vi "FeedbackDecode_PickROI_Adv.vi"(3 "RespStrRef":refnum<vi>) -> ()   [LabVIEW 2020]
uses:
  <vilib>/Utility/miscctls.llb/LVPoint32TypeDef.ctl
  FeedbackDecode_Globals.vi
  <vilib>/imath/engines/lvmath2/RunTimeEngine/IndexRead/NIMS M($,S).vi
  <instcachedir>/0/NIMS M($,S)_3E5749BBB62E49528D4765A77F1F6D98.lvgen/NIMS M($,S)_3E5749BBB62E49528D4765A77F1F6D98_000.vi
  <vilib>/imath/engines/lvmath2/RunTimeEngine/IndexRead/NIMS V(S).vi
  <instcachedir>/0/NIMS V(S)_0488751826AF41519A22953C041130DC.lvgen/NIMS V(S)_0488751826AF41519A22953C041130DC_000.vi
  <vilib>/imath/engines/lvmath2/RunTimeEngine/BuiltInFunctions/abs/NIMS_abs(signed).vi
  <instcachedir>/0/NIMS_abs(signed)_C4FCB8E6058B49B797C7C8D53CA5F6EC.lvgen/NIMS_abs(signed)_C4FCB8E6058B49B797C7C8D53CA5F6EC_001.vi
  <vilib>/imath/engines/lvmath2/RunTimeEngine/IndexReplace/NIMS M($,S)=V.vi
  <instcachedir>/0/NIMS M($,S)=V_85A28EB895514E96A13A10261726EE3A.lvgen/NIMS M($,S)=V_85A28EB895514E96A13A10261726EE3A_001.vi
  <vilib>/imath/engines/lvmath2/RunTimeEngine/ErrorHandling/NIMS_Create Error From Enums.vi
  <vilib>/imath/engines/lvmath2/RunTimeEngine/BuiltInFunctions/sum/NIMS_sum(GM,Sca).vi
  <instcachedir>/0/NIMS_sum(GM,Sca)_BFF867FCA20B40888962313BF0DBA2C0.lvgen/NIMS_sum(GM,Sca)_BFF867FCA20B40888962313BF0DBA2C0_001.vi
  <vilib>/imath/engines/lvmath2/RunTimeEngine/BuiltInFunctions/min/1 input/NIMS_min(RV).vi
  <instcachedir>/0/NIMS_min(RV)_EE2DD3E2888846108C5160A664B67832.lvgen/NIMS_min(RV)_EE2DD3E2888846108C5160A664B67832_000.vi
  <vilib>/imath/engines/lvmath2/RunTimeEngine/NodeEndStatement/NIMS_NodeEndStatement_Output.vi
  <instcachedir>/0/NIMS_NodeEndStatement_Output_53EC0D466D134D7ABD903AC30B43404B.lvgen/NIMS_NodeEndStatement_Output_53EC0D466D134D7ABD903AC30B43404B_010.vi
  <vilib>/imath/engines/lvmath2/RunTimeEngine/ErrorHandling/NIMS_Finalize Error.vi
panel:
  out "RegionStr":string
  out "SensorStr":string
  out "Description_array":string[](array[string])
  out "CursClck":dbl[](array[numeric])
  in  "Advance":bool
  out "StepAdvnc":dbl
  out "Perception_array":string[](array[string])
  out "Sensor_array":string[][](array[string])
  out "Region_array":string[][](array[string])
  out "Y_array":dbl[][](array[numeric])
  out "X_array":dbl[][](array[numeric])
  out "Sensor":string[](array[string])
  out "Region":string[](array[string])
  out "Xcoord":dbl[](array[numeric])
  out "Ycoord":dbl[](array[numeric])
  out "Palette":u32[](array[colorbox])=[16711680, 15697664, 16772882, 8584960, 61382, 14847, 11534591]
  out "CrcColor":u32=16711680
  out "PPath2":path=path "C:/Users/Administrator/Code/Tasks/FeedbackDecode/resources/RightHand_region_colored.jpg"
  in  "DscrptnBtns":T1
  in  "ClearRsp":bool
  in  "PerceptBtns":T2
  out "PickROIStr":string
  in  "Array 4":string[][](array[string])
  out "RegionStr":string[][](array[string])=[["G1", "1", "231", "255", "231", "T1", "", ""], ["G2", "2", "201", "254", "200", "T2", "", ""], ["G3", "3", "211", "235", "211", "T3", "", ""], ["G4", "4", "188", "236", "188", "T4", "", ""], ["G5", "5", "141", "235", "141", "T5", "", ""], ["G6", "6", "164", "235", "165", "T6", "", ""], ["G7", "7", "117", "234", "117", "P1", "", ""], ["G8", "8", "70", "235", "70", "P6", "", ""], ["G9", "9", "94", "235", "94", "P9", "", ""], ["G10", "10", "46", "235", "47", "P7", "", ""], ["G11", "11", "3", "235", "3", "P8", "", ""], ["G12", "12", "23", "236", "24", "P10", "", ""], ["R1", "13", "248", "200", "200", "I1", "", ""], ["R2", "14", "248", "180", "181", "I2", "", ""], ["R3", "15", "248", "150", "151", "I3", "", ""], ["R4", "16", "248", "120", "121", "I4", "", ""], ["R5", "17", "248", "100", "100", "I5", "", ""], ["R6", "18", "248", "80", "80", "I6", "", ""], ["R7", "19", "248", "60", "61", "I7", "", ""], ["R8", "20", "248", "30", "29", "I8", "", ""], ["R9", "21", "247", "2", "2", "P2", "", ""], ["O1", "22", "243", "210", "195", "M1", "", ""], ["O2", "23", "244", "194", "171", "M2", "", ""], ["O3", "24", "243", "178", "145", "M3", "", ""], ["O4", "25", "244", "162", "122", "M4", "", ""], ["O5", "26", "243", "145", "98", "M5", "", ""], ["O6", "27", "244", "129", "74", "M6", "", ""], ["O7", "28", "243", "113", "48", "M7", "", ""], ["O8", "29", "243", "97", "24", "M8", "", ""], ["O9", "30", "243", "80", "0", "P3", "", ""], ["Y1", "31", "232", "225", "209", "R1", "", ""], ["Y2", "32", "232", "218", "187", "R2", "", ""], ["Y3", "33", "232", "210", "163", "R3", "", ""], ["Y4", "34", "230", "205", "138", "R4", "", ""], ["Y5", "35", "233", "196", "116", "R5", "", ""], ["Y6", "36", "232", "187", "93", "R6", "", ""], ["Y7", "37", "233", "181", "71", "R7", "", ""], ["Y8", "38", "232", "173", "47", "R8", "", ""], ["Y9", "39", "232", "159", "0", "P4", "", ""], ["YG1", "40", "213", "232", "186", "L1", "", ""], ["YG2", "41", "202", "232", "162", "L2", "", ""], ["YG3", "42", "193", "232", "139", "L3", "", ""], ["YG4", "43", "182", "232", "117", "L4", "", ""], ["YG5", "44", "171", "232", "93", "L5", "", ""], ["YG6", "45", "161", "231", "70", "L6", "", ""], ["YG7", "46", "152", "232", "47", "L7", "", ""], ["YG8", "47", "142", "232", "23", "L8", "", ""], ["YG9", "48", "130", "234", "0", "P5", "", ""], ["P1", "49", "250", "227", "253", "DT1", "", ""], ["P2", "50", "245", "203", "253", "DT2", "", ""], ["P3", "51", "241", "177", "253", "DT3", "", ""], ["P4", "52", "238", "152", "253", "DT4", "", ""], ["P5", "53", "235", "126", "253", "DT5", "", ""], ["P6", "54", "230", "101", "253", "DT6", "", ""], ["P7", "55", "227", "76", "253", "D1", "", ""], ["P8", "56", "223", "50", "253", "D6", "", ""], ["P9", "57", "220", "25", "253", "D9", "", ""], ["P10", "58", "215", "0", "254", "D7", "", ""], ["P11", "59", "167", "0", "254", "D8", "", ""], ["P12", "60", "188", "52", "255", "D10", "", ""], ["BG1", "61", "204", "240", "234", "DI1", "", ""], ["BG2", "62", "168", "240", "226", "DI2", "", ""], ["BG3", "63", "144", "240", "221", "DI3", "", ""], ["BG4", "64", "120", "240", "216", "DI4", "", ""], ["BG5", "65", "96", "240", "211", "DI5", "", ""], ["BG6", "66", "72", "240", "206", "DI6", "", ""], ["BG7", "67", "48", "240", "202", "DI7", "", ""], ["BG8", "68", "24", "240", "197", "DI8", "", ""], ["BG9", "69", "0", "240", "192", "D2", "", ""], ["LB1", "70", "186", "229", "232", "DM1", "", ""], ["LB2", "71", "163", "228", "232", "DM2", "", ""], ["LB3", "72", "139", "226", "232", "DM3", "", ""], ["LB4", "73", "116", "225", "232", "DM4", "", ""], ["LB5", "74", "93", "223", "232", "DM5", "", ""], ["LB6", "75", "70", "222", "232", "DM6", "", ""], ["LB7", "76", "46", "220", "232", "DM7", "", ""], ["LB8", "77", "23", "218", "232", "DM8", "", ""], ["LB9", "78", "0", "217", "232", "D3", "", ""], ["B1", "79", "204", "224", "255", "DR1", "", ""], ["B2", "80", "179", "208", "255", "DR2", "", ""], ["B3", "81", "153", "192", "255", "DR3", "", ""], ["B4", "82", "127", "177", "255", "DR4", "", ""], ["B5", "83", "103", "161", "255", "DR5", "", ""], ["B6", "84", "76", "145", "255", "DR6", "", ""], ["B7", "85", "52", "129", "255", "DR7", "", ""], ["B8", "86", "25", "113", "255", "DR8", "", ""], ["B9", "87", "0", "96", "255", "D4", "", ""], ["BP1", "88", "230", "230", "255", "DL1", "", ""], ["BP2", "89", "180", "179", "255", "DL2", "", ""], ["BP3", "90", "155", "153", "255", "DL3", "", ""], ["BP4", "91", "130", "127", "255", "DL4", "", ""], ["BP5", "92", "105", "103", "255", "DL5", "", ""], ["BP6", "93", "79", "76", "255", "DL6", "", ""], ["BP7", "94", "54", "52", "255", "DL7", "", ""], ["BP8", "95", "29", "25", "255", "DL8", "", ""], ["BP9", "96", "6", "0", "255", "D5", "", ""]]
  in  "Array 3":dbl[][](array[numeric])
  out "RGB 2":dbl[](array[numeric])=[92.0, 223.0, 233.0]
  out "RGBtbl 2":dbl[][](array[numeric])=[[231.0, 255.0, 231.0], [201.0, 254.0, 200.0], [211.0, 235.0, 211.0], [188.0, 236.0, 188.0], [141.0, 235.0, 141.0], [164.0, 235.0, 165.0], [117.0, 234.0, 117.0], [70.0, 235.0, 70.0], [94.0, 235.0, 94.0], [46.0, 235.0, 47.0], [3.0, 235.0, 3.0], [23.0, 236.0, 24.0], [248.0, 200.0, 200.0], [248.0, 180.0, 181.0], [248.0, 150.0, 151.0], [248.0, 120.0, 121.0], [248.0, 100.0, 100.0], [248.0, 80.0, 80.0], [248.0, 60.0, 61.0], [248.0, 30.0, 29.0], [247.0, 2.0, 2.0], [243.0, 210.0, 195.0], [244.0, 194.0, 171.0], [243.0, 178.0, 145.0], [244.0, 162.0, 122.0], [243.0, 145.0, 98.0], [244.0, 129.0, 74.0], [243.0, 113.0, 48.0], [243.0, 97.0, 24.0], [243.0, 80.0, 0.0], [232.0, 225.0, 209.0], [232.0, 218.0, 187.0], [232.0, 210.0, 163.0], [230.0, 205.0, 138.0], [233.0, 196.0, 116.0], [232.0, 187.0, 93.0], [233.0, 181.0, 71.0], [232.0, 173.0, 47.0], [232.0, 159.0, 0.0], [213.0, 232.0, 186.0], [202.0, 232.0, 162.0], [193.0, 232.0, 139.0], [182.0, 232.0, 117.0], [171.0, 232.0, 93.0], [161.0, 231.0, 70.0], [152.0, 232.0, 47.0], [142.0, 232.0, 23.0], [130.0, 234.0, 0.0], [250.0, 227.0, 253.0], [245.0, 203.0, 253.0], [241.0, 177.0, 253.0], [238.0, 152.0, 253.0], [235.0, 126.0, 253.0], [230.0, 101.0, 253.0], [227.0, 76.0, 253.0], [223.0, 50.0, 253.0], [220.0, 25.0, 253.0], [215.0, 0.0, 254.0], [167.0, 0.0, 254.0], [188.0, 52.0, 255.0], [204.0, 240.0, 234.0], [168.0, 240.0, 226.0], [144.0, 240.0, 221.0], [120.0, 240.0, 216.0], [96.0, 240.0, 211.0], [72.0, 240.0, 206.0], [48.0, 240.0, 202.0], [24.0, 240.0, 197.0], [0.0, 240.0, 192.0], [186.0, 229.0, 232.0], [163.0, 228.0, 232.0], [139.0, 226.0, 232.0], [116.0, 225.0, 232.0], [93.0, 223.0, 232.0], [70.0, 222.0, 232.0], [46.0, 220.0, 232.0], [23.0, 218.0, 232.0], [0.0, 217.0, 232.0], [204.0, 224.0, 255.0], [179.0, 208.0, 255.0], [153.0, 192.0, 255.0], [127.0, 177.0, 255.0], [103.0, 161.0, 255.0], [76.0, 145.0, 255.0], [52.0, 129.0, 255.0], [25.0, 113.0, 255.0], [0.0, 96.0, 255.0], [230.0, 230.0, 255.0], [180.0, 179.0, 255.0], [155.0, 153.0, 255.0], [130.0, 127.0, 255.0], [105.0, 103.0, 255.0], [79.0, 76.0, 255.0], [54.0, 52.0, 255.0], [29.0, 25.0, 255.0], [6.0, 0.0, 255.0]]
  out "Resample 2":bool=TRUE
  out "Count 2":i32
  out "ErMsg 2":bool
  out "2D Picture 2":picture
  out "Coords":T3={"Horizontal"=176, "Vertical"=80}
  out "Output Color":u32(colorbox)=6086633
  in  "Abort":bool
  out "Click":bool
  out "RGBtbl":dbl[][](array[numeric])=[[236.0, 28.0, 36.0], [216.0, 207.0, 255.0], [249.0, 136.0, 49.0], [165.0, 255.0, 153.0], [249.0, 189.0, 49.0], [236.0, 236.0, 28.0], [52.0, 28.0, 236.0], [170.0, 28.0, 236.0], [236.0, 28.0, 174.0], [255.0, 170.0, 230.0], [140.0, 255.0, 251.0], [27.0, 234.0, 189.0], [25.0, 178.0, 89.0]]
  in  "Array 2":dbl[][](array[numeric])
  out "SensStr":string[][](array[string])=[["Red", "1", "236", "28", "36", "thumb_distal"], ["Lavender", "2", "216", "207", "255", "thumb_distal"], ["Orange", "3", "249", "136", "49", "palm_back"], ["LGreen", "4", "165", "255", "153", "palm_side"], ["Gold", "5", "249", "189", "49", "palm_thumb"], ["Yellow", "6", "236", "236", "28", "palm_pinky"], ["Blue", "7", "52", "28", "236", "pinky_distal"], ["Purple", "8", "170", "28", "236", "ring_distal"], ["Magenta", "9", "236", "28", "174", "middle_distal"], ["Pink", "10", "255", "170", "230", "index_distal"], ["LBlue", "11", "140", "255", "251", "index_medial"], ["BGreen", "12", "27", "234", "189", "thumb_distal"], ["Green", "13", "25", "178", "89", "thumb_medial"]]
  in  "Array":string[][](array[string])
  out "ErMsg":bool
  out "Count":i32=5
  out "Resample":bool
  out "RGB":dbl[](array[numeric])=[255.0, 255.0, 255.0]
  out "2D Picture":picture
  in  "Submit":bool
  # "1. Click on the region(s) where the sensation occurs :"
  # "2. Describe the sensation (choose one):"
  # "3. Choose between each pair:"
  # "4. Describe another \nsensation (optional):"
  # "5. Submit response:"
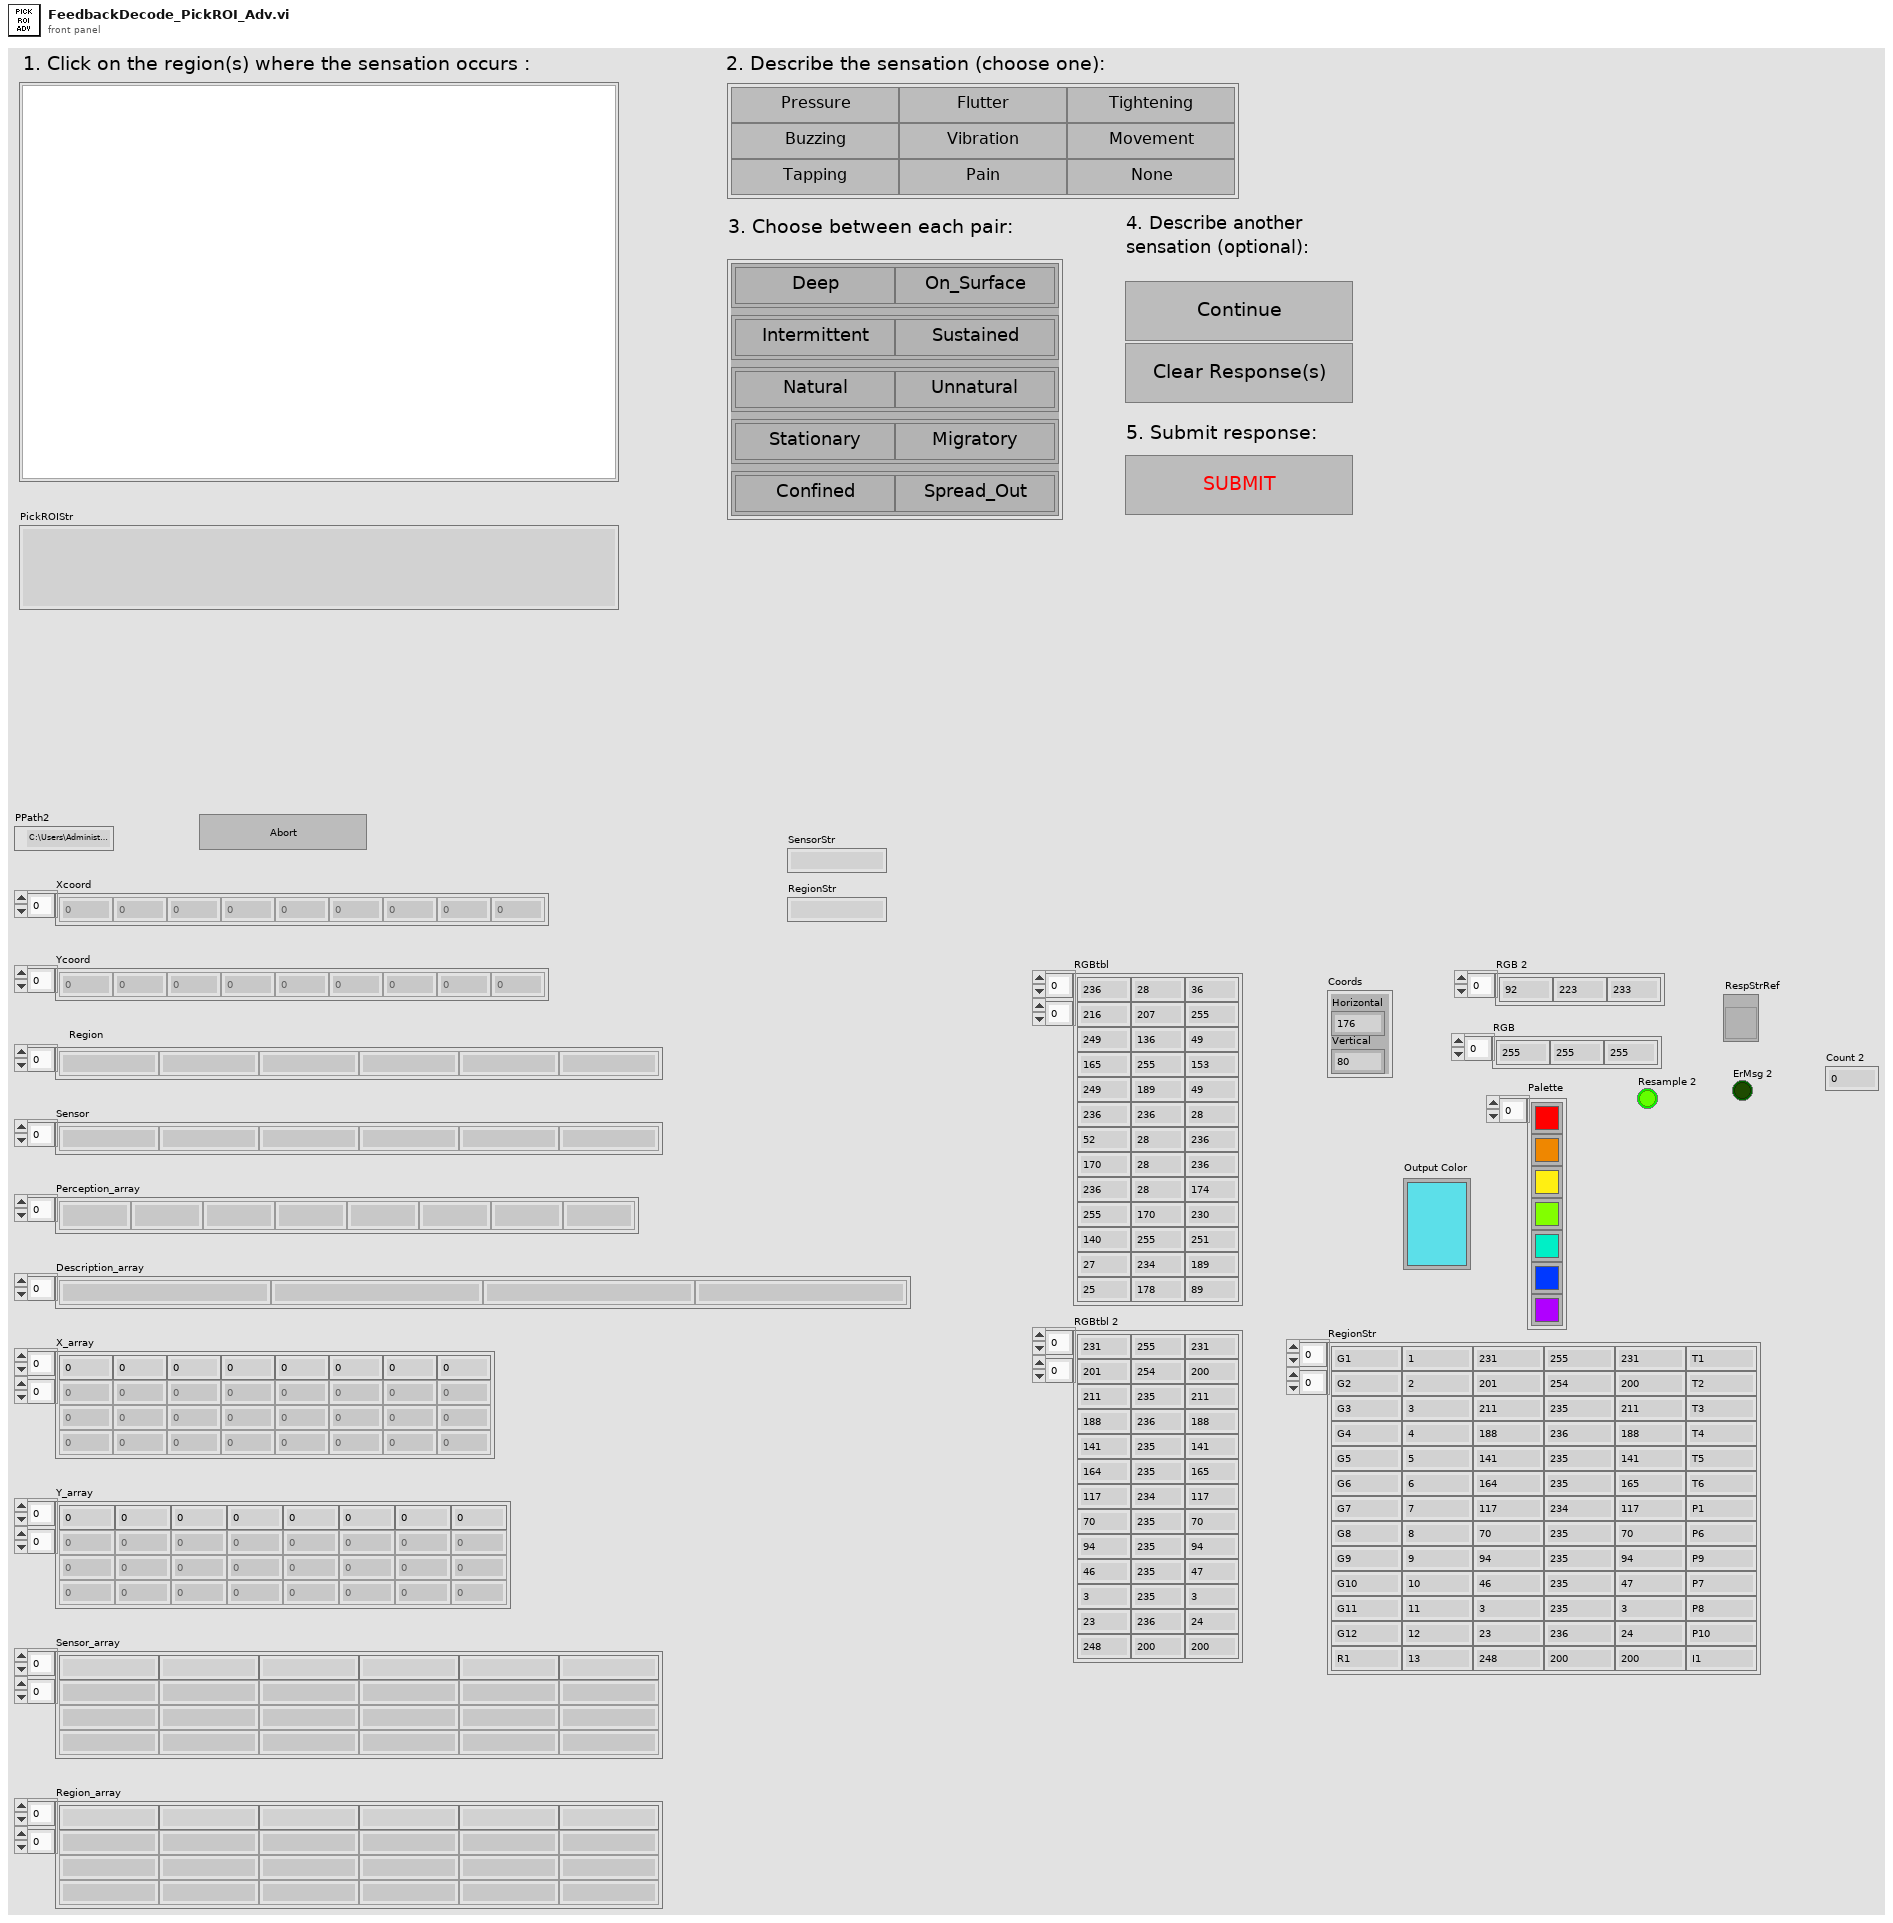
[diagram p1: front panel]
types:
  T1 = cluster{"2afc 3":cluster{"Stationary":bool, "Migratory":bool}, "2afc 2":cluster{"Natural":bool, "Unnatural":bool}, "2afc 4":cluster{"Confined":bool, "Spread":bool}, "2afc 1":cluster{"Intermittent":bool, "Sustained":bool}, "2afc 0":cluster{"Deep":bool, "Surface":bool}}
  T2 = cluster{"Buzzing":bool, "Pressure":bool, "Tapping":bool, "None":bool, "Flutter":bool, "Vibration":bool, "Pain":bool, "Tightening":bool, "Movement":bool}
  T3 = typedef "LVPoint32TypeDef.ctl" = cluster{"Horizontal":i32, "Vertical":i32}
  T4 = cluster{"Motion":bool, "Pressure":bool, "Tapping":bool, "None":bool, "Flutter":bool, "Vibration":bool, "Pain":bool, "Tightening":bool, "Movement":bool}
  T5 = typedef "imagedata.ctl" = cluster{"image type":i32, "image depth":i32, "image":u8[], "mask":u8[], "colors":u32[], "Rectangle":cluster{"left":i16, "top":i16, "right":i16, "bottom":i16}}
  T6 = typedef "LVPositionTypeDef.ctl" = cluster{"Left":i32, "Top":i32}
  T7 = enum32{"Invalid", "Standard", "Closed", "Hidden", "Minimized", "Maximized"}
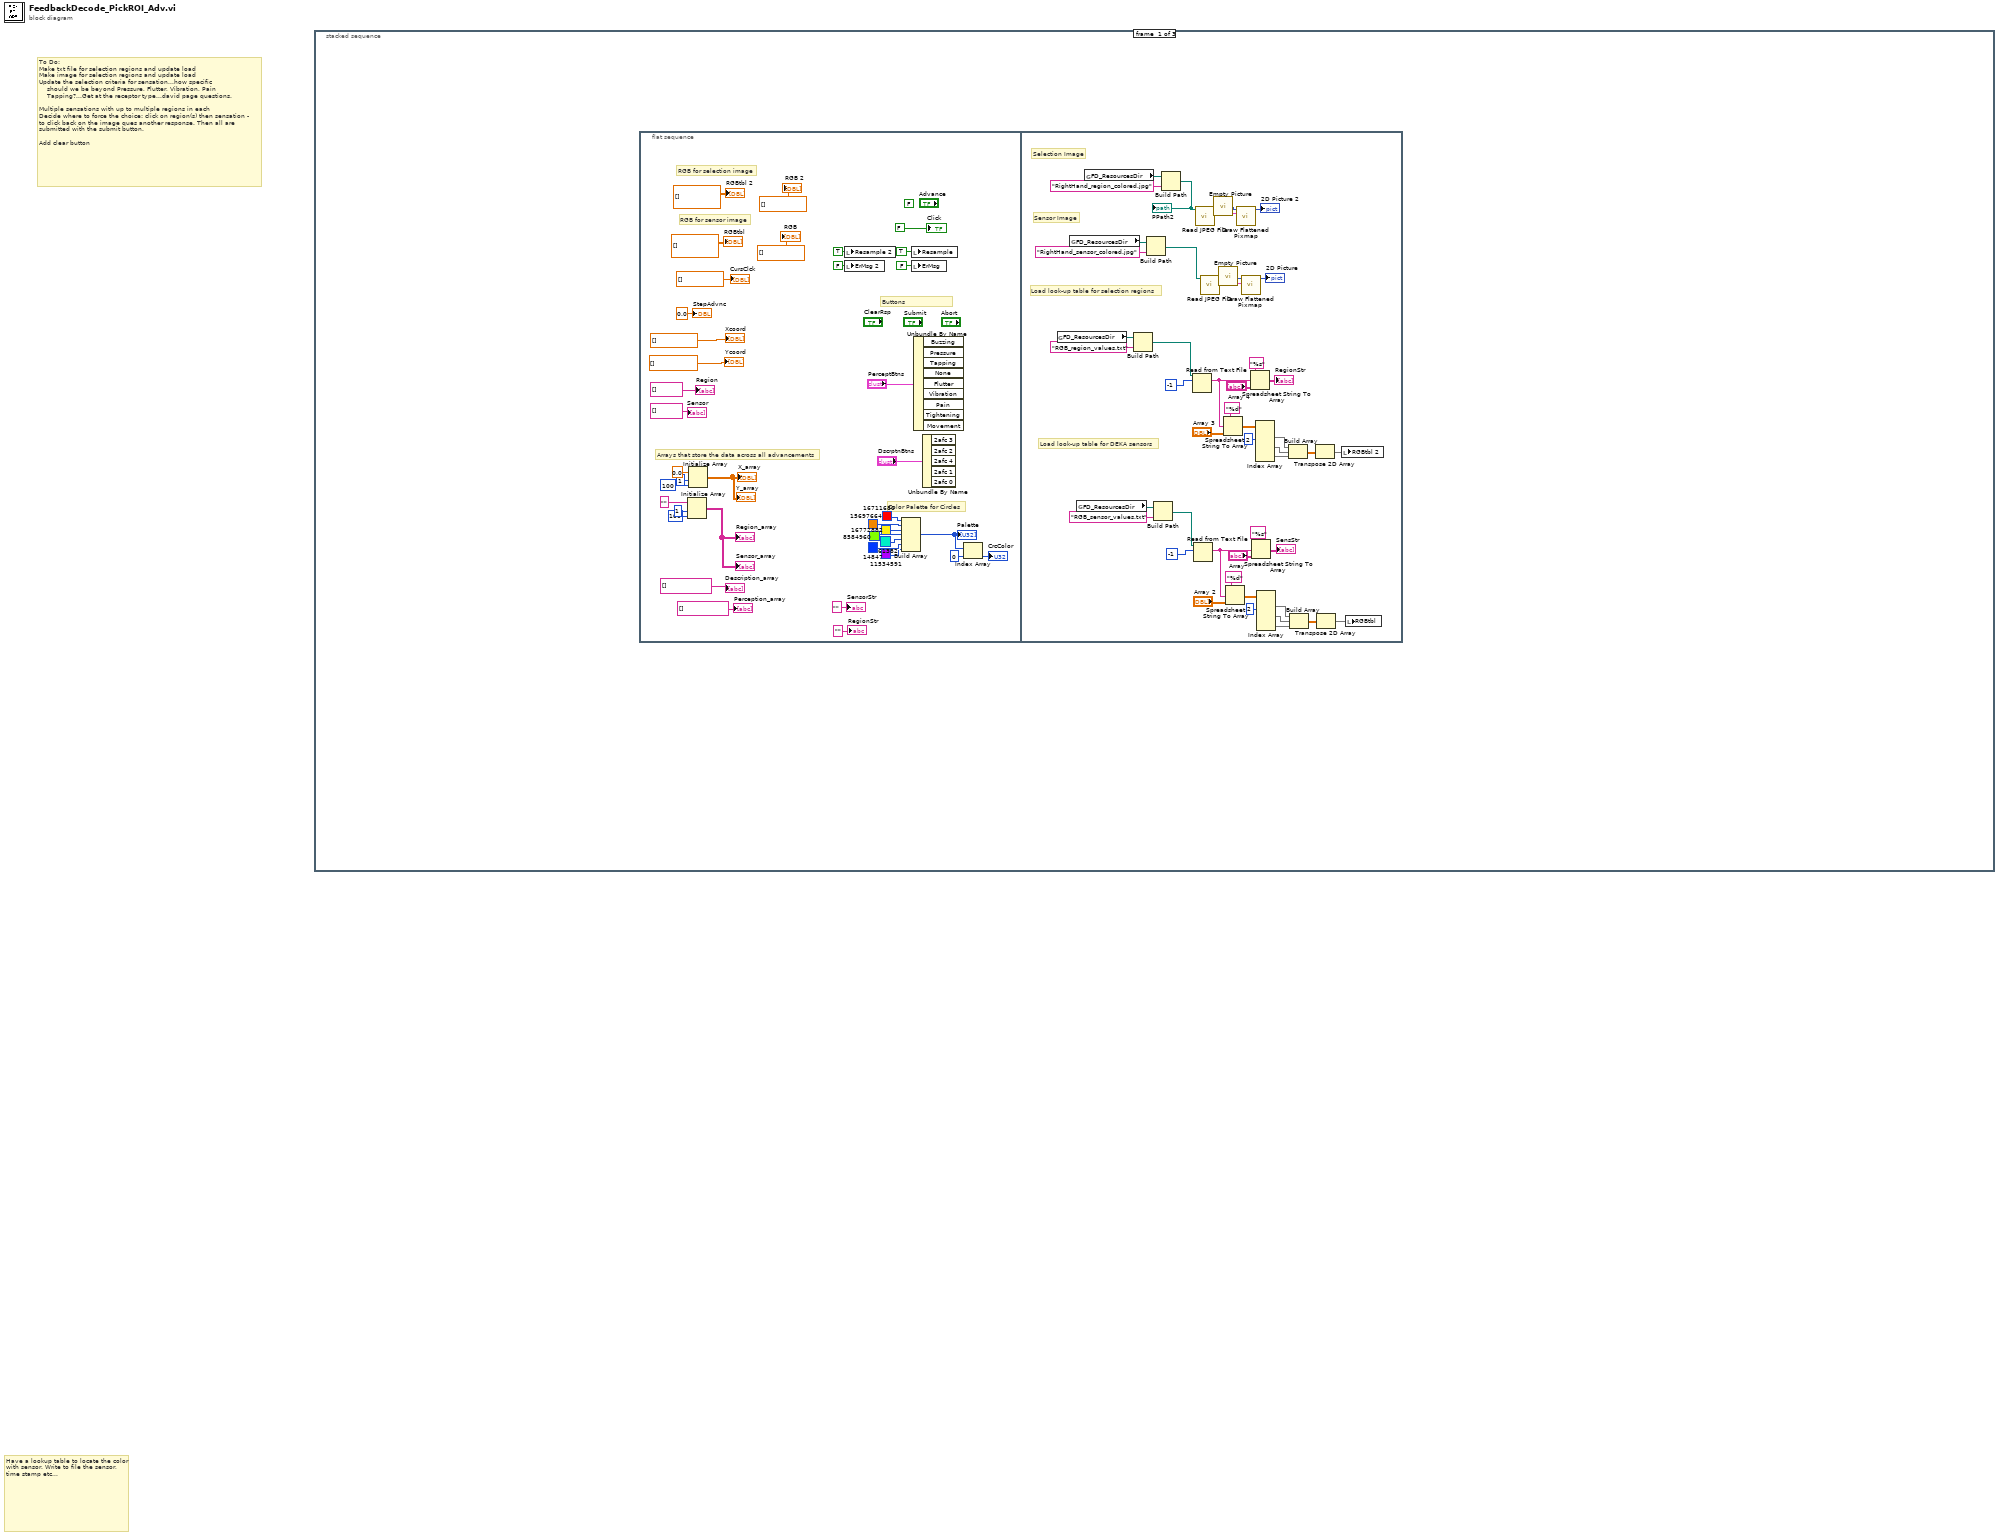
[diagram p0: block diagram]
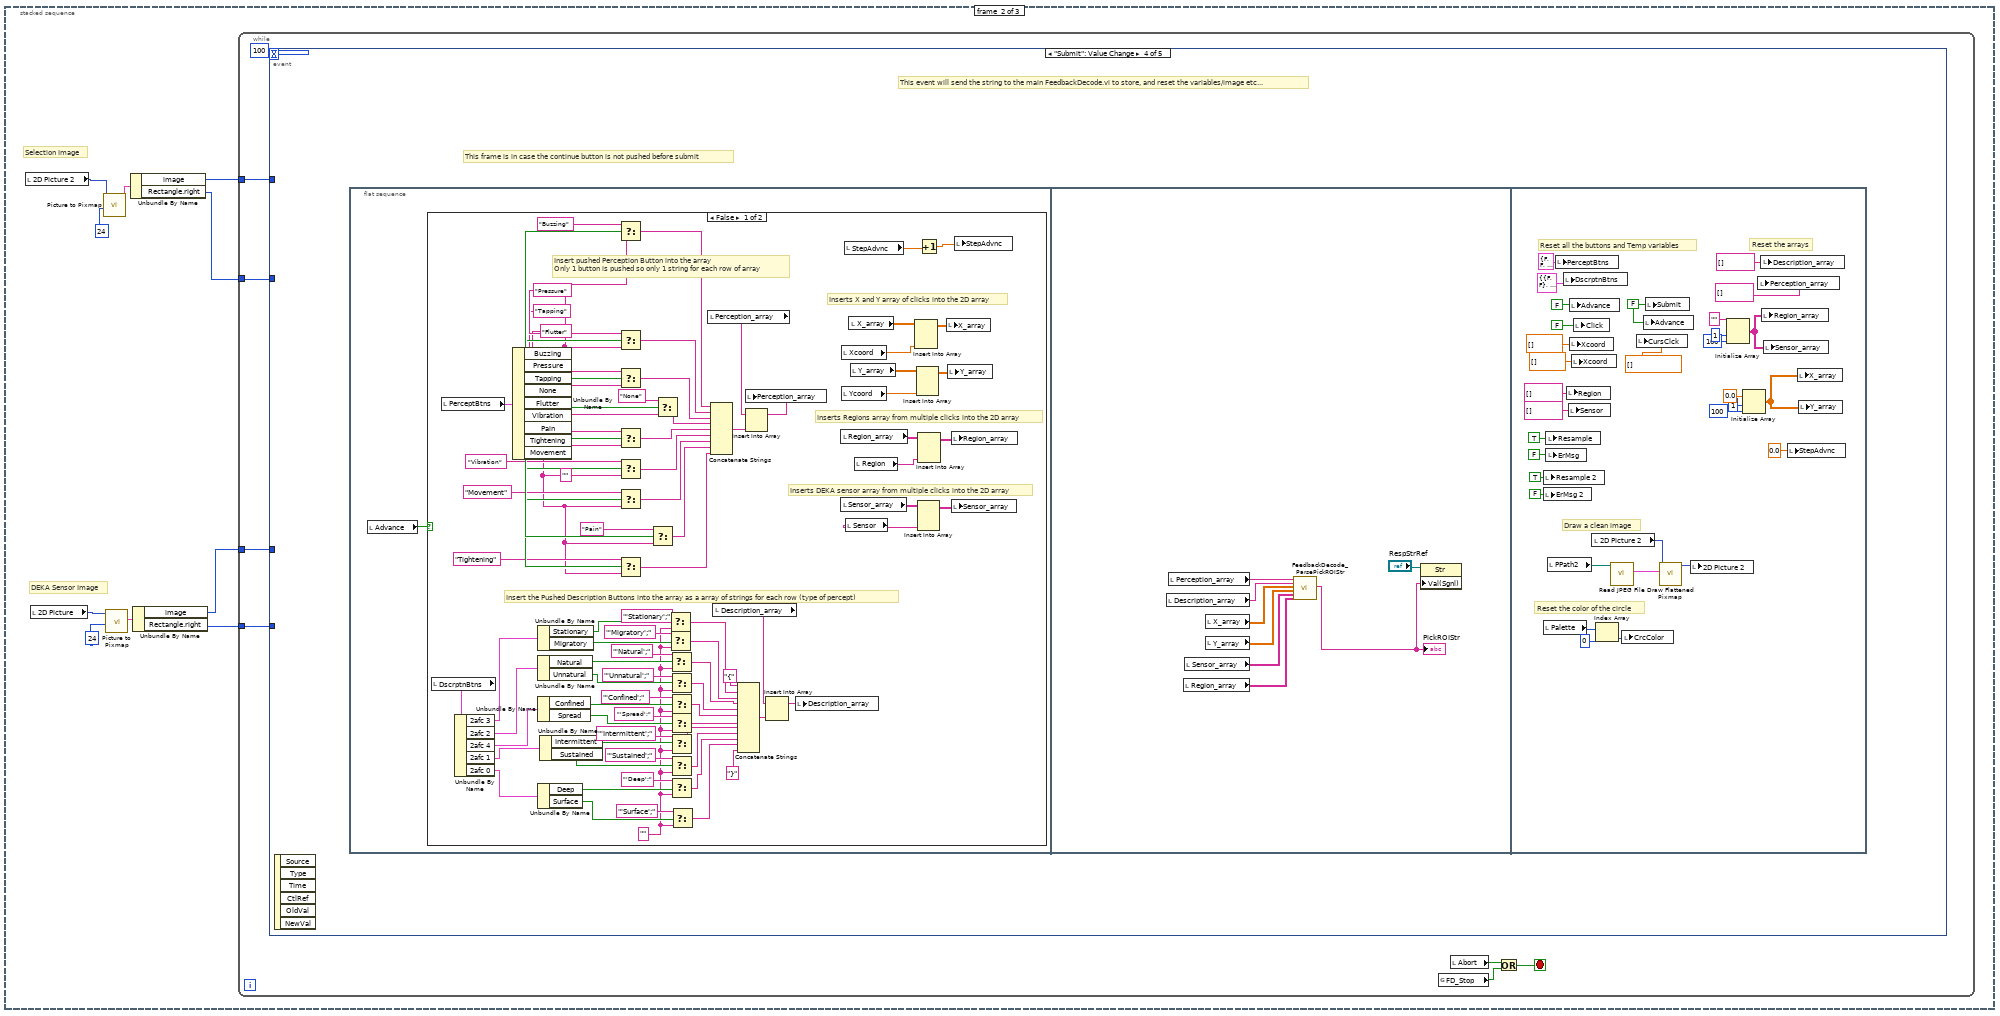
[diagram p2: hidden frame]
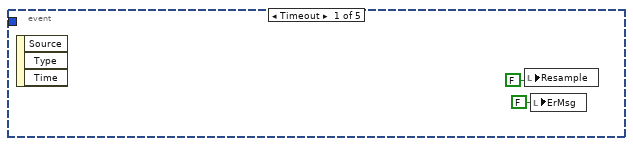
[diagram p3: hidden frame]
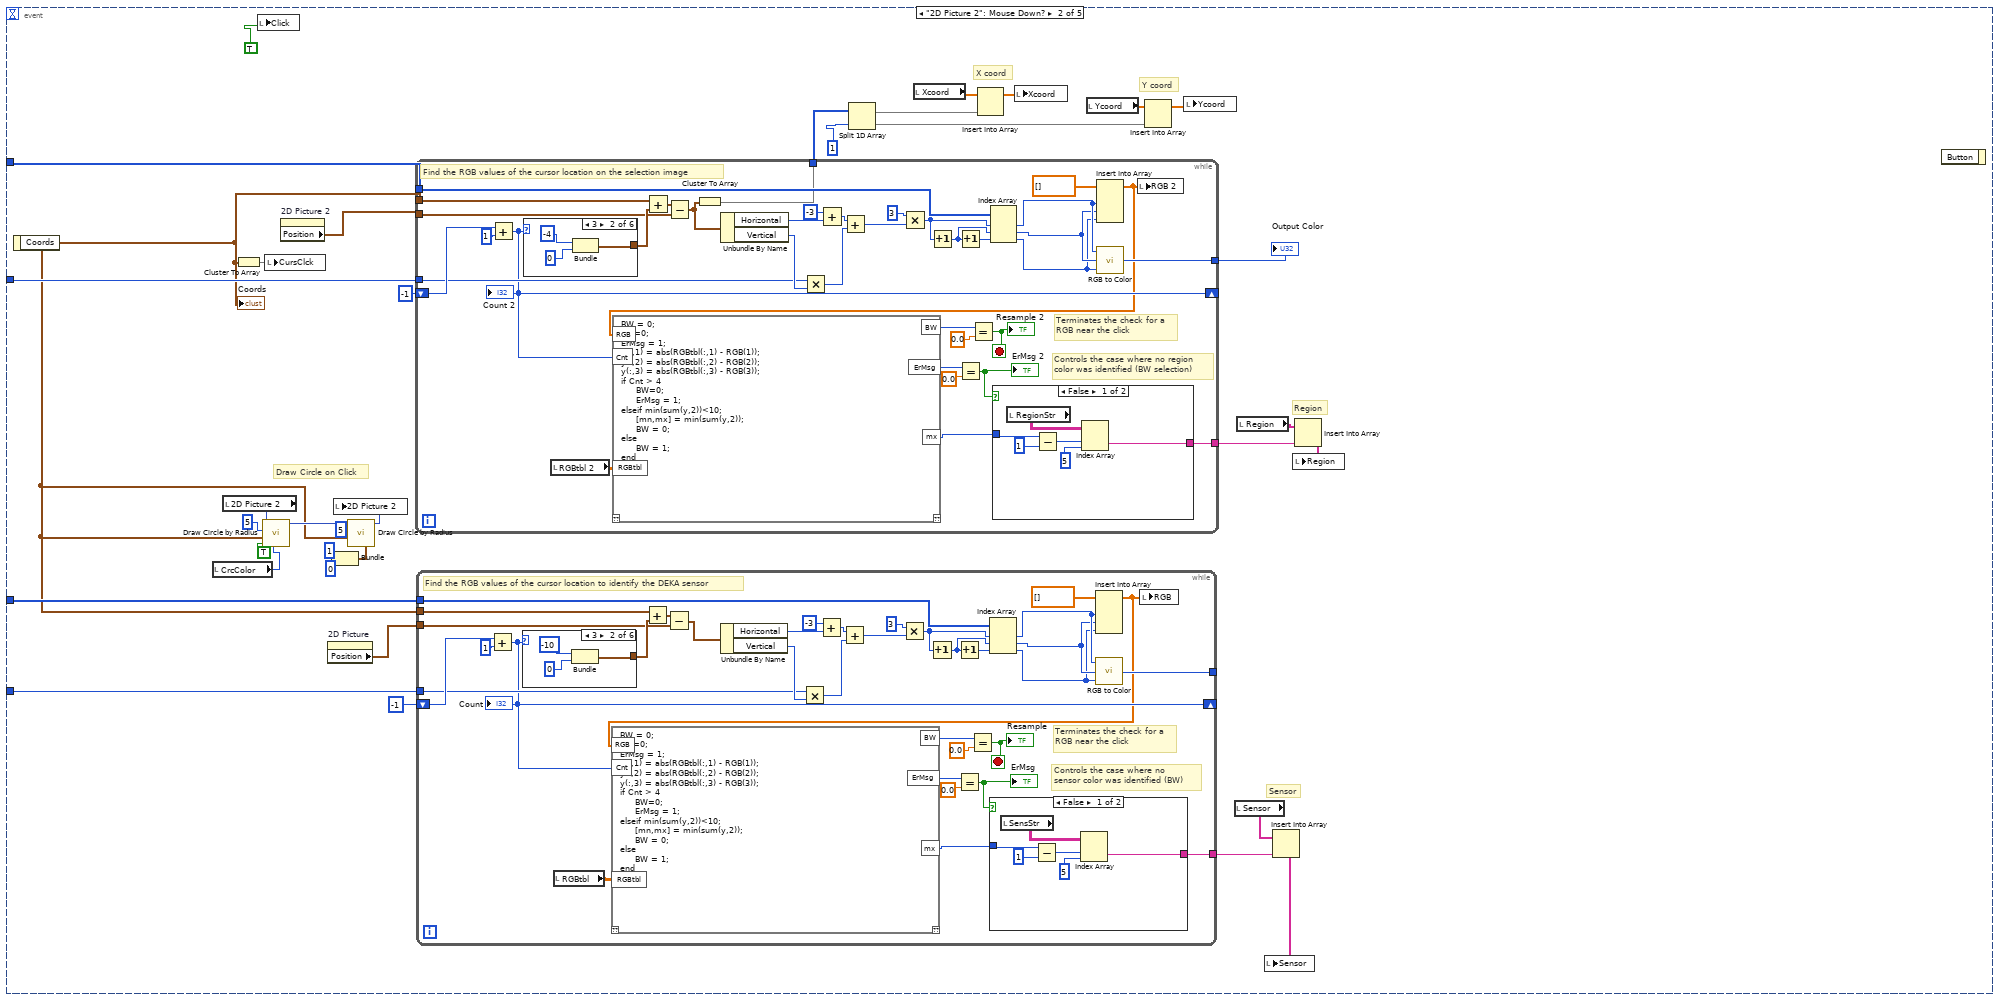
[diagram p4: hidden frame]
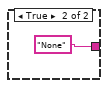
[diagram p5: hidden frame]
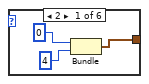
[diagram p6: hidden frame]
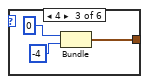
[diagram p7: hidden frame]
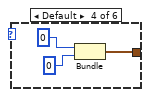
[diagram p8: hidden frame]
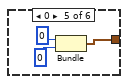
[diagram p9: hidden frame]
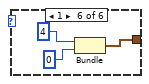
[diagram p10: hidden frame]
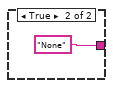
[diagram p11: hidden frame]
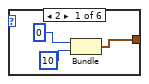
[diagram p12: hidden frame]
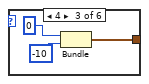
[diagram p13: hidden frame]
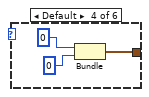
[diagram p14: hidden frame]
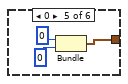
[diagram p15: hidden frame]
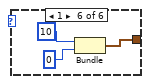
[diagram p16: hidden frame]
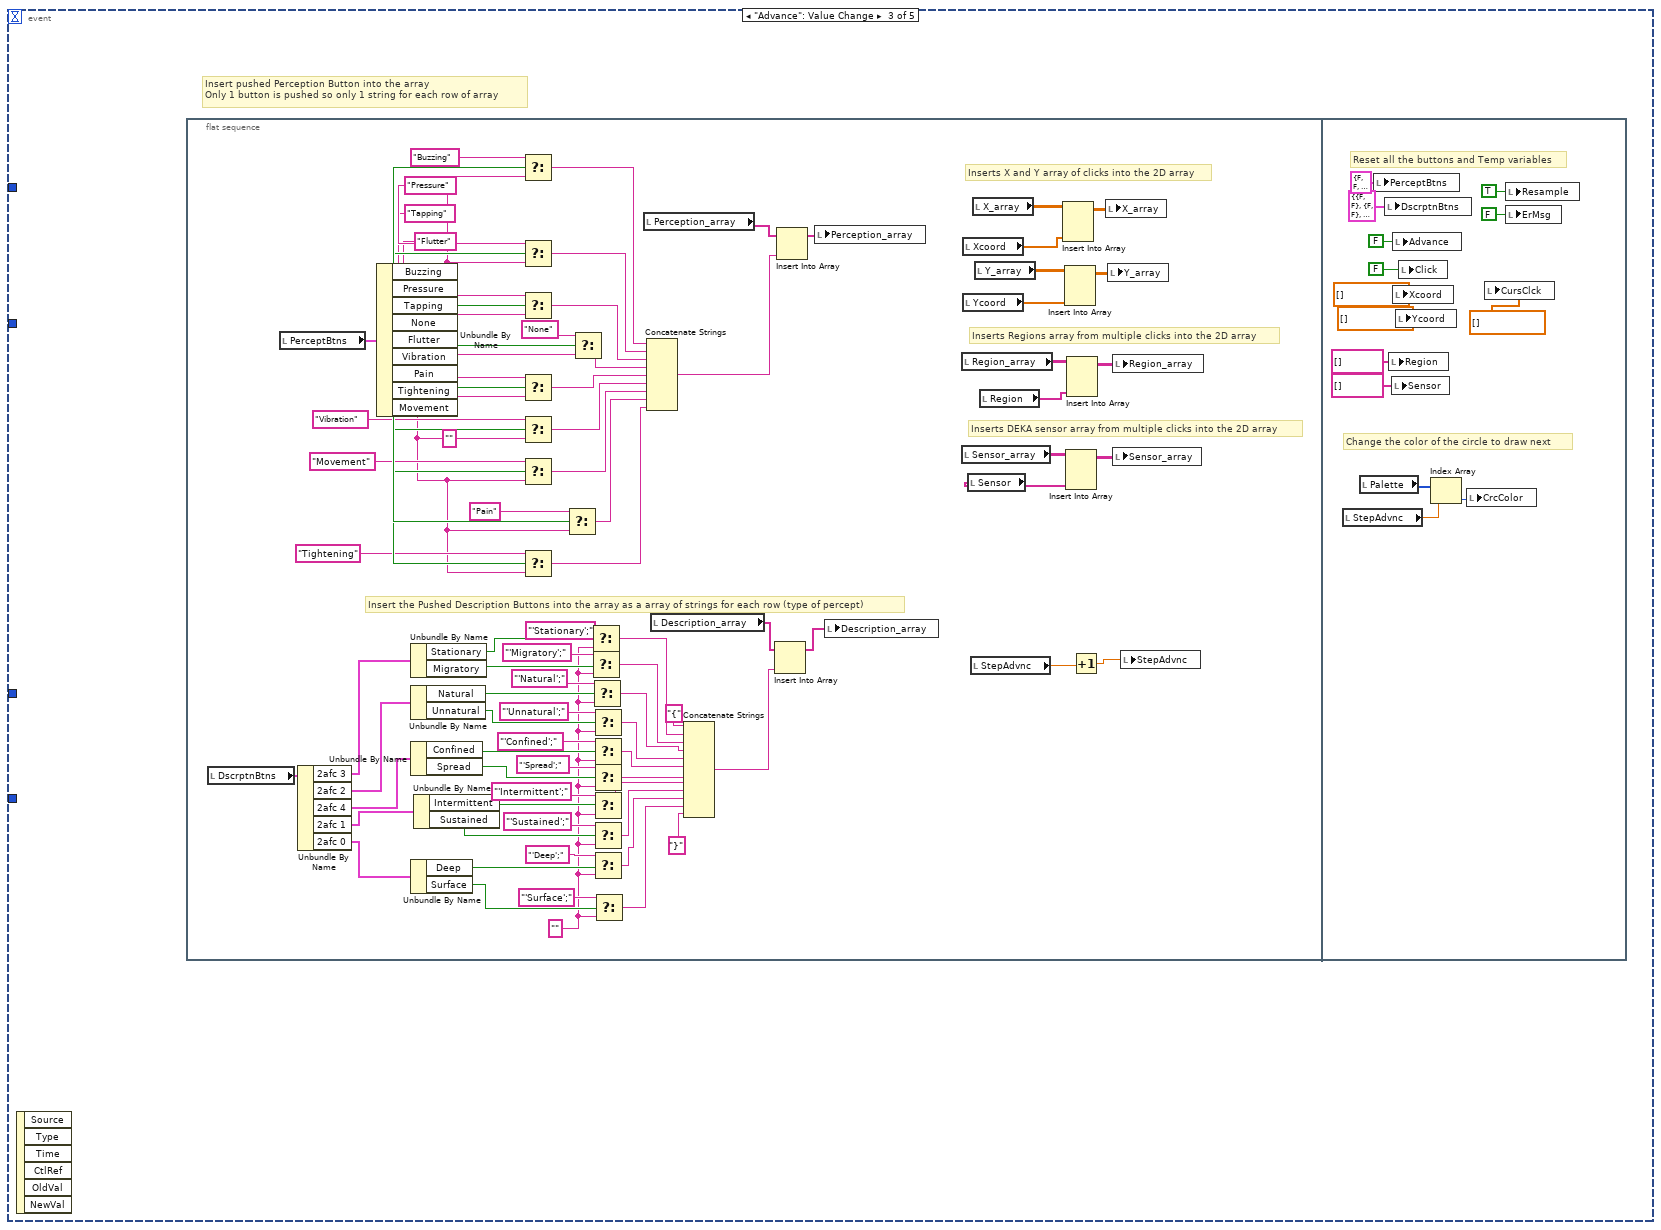
[diagram p17: hidden frame]
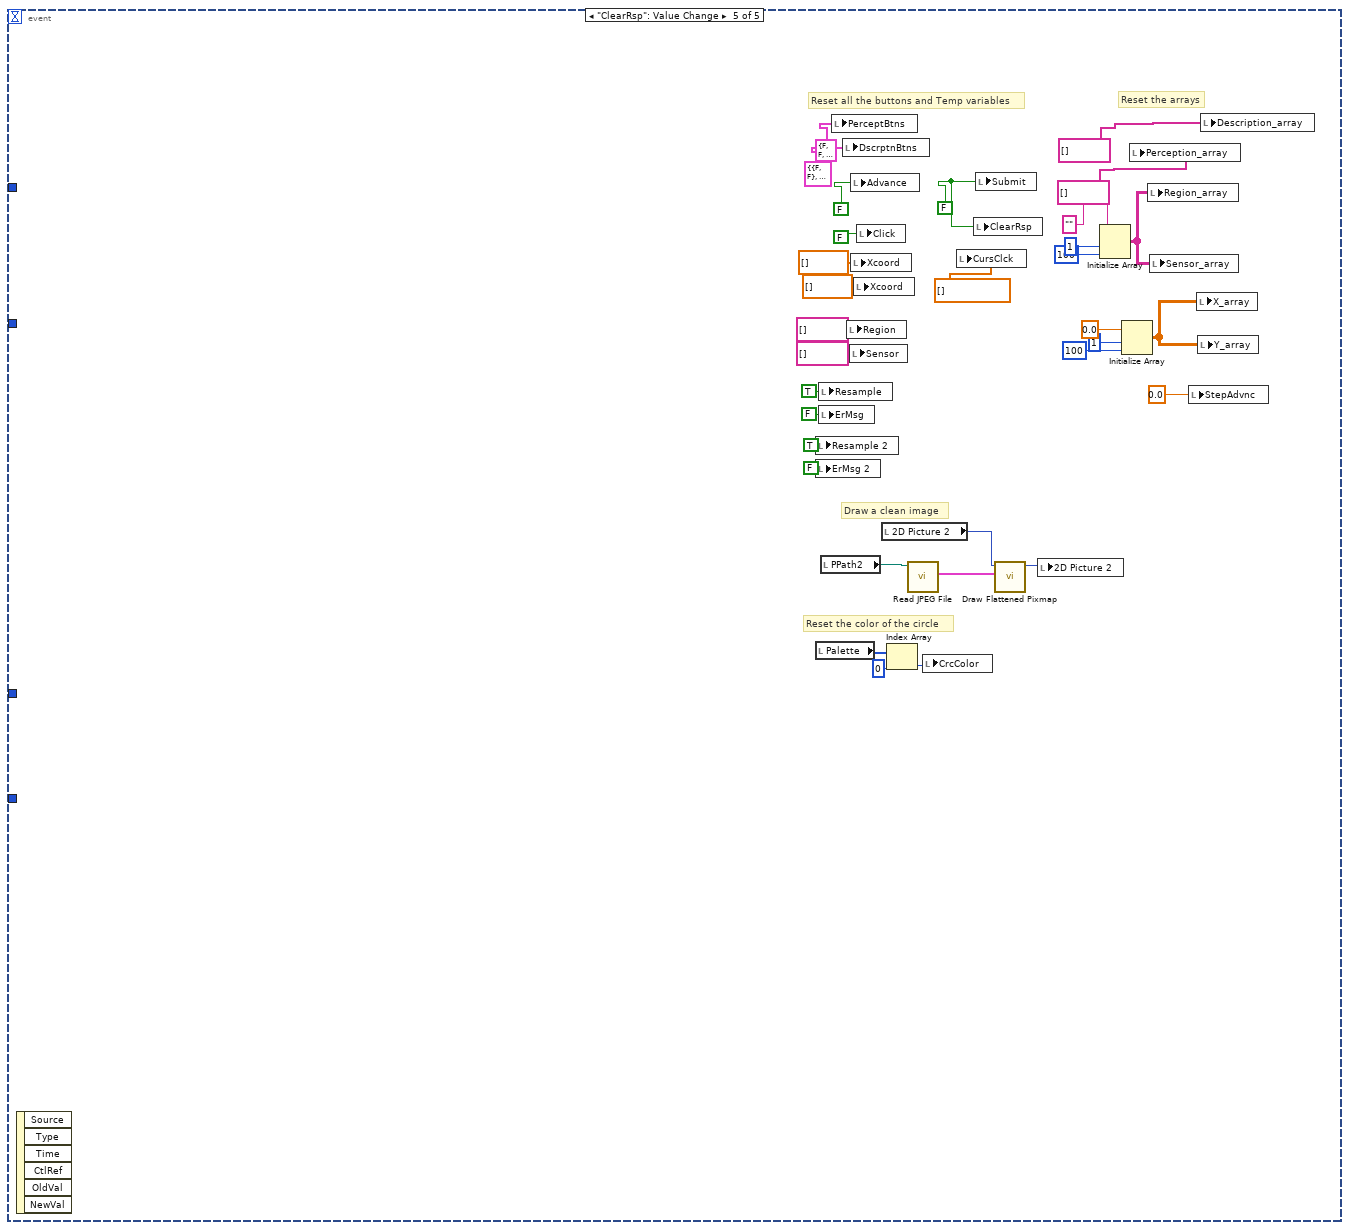
[diagram p19: hidden frame]
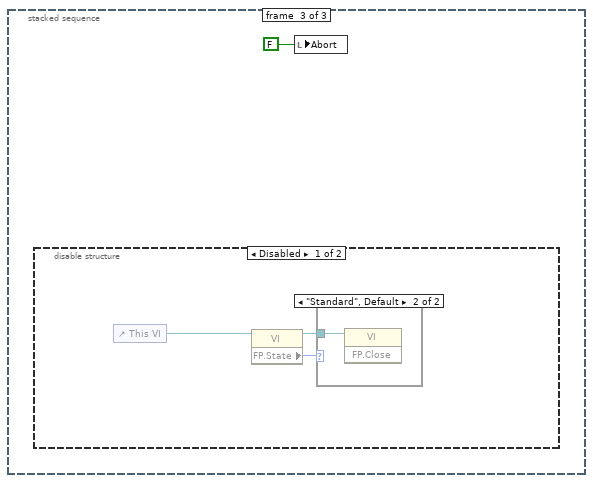
[diagram p20: hidden frame]
diagram:
  # "To Do:\nMake txt file for selection regions and update load\nMake image for selection regions and update load\nUpdate the selection criteria for sensation...how specific\n    should we be beyond Pressure, Flutter, Vibration, Pain\n    Tapping?...Get at the receptor type...david page questions.\n\nMultiple sensations with up to multiple regions in each\nDecide where to force the choice: click on region(s) then sensation - \nto click back on the image ques another response. Then all are\nsubmitted with the submit button.\n\nAdd clear button"
  # "Have a lookup table to locate the color with sensor. Write to file the sensor, time stamp etc..."
  n1 = stacked-sequence {
    frame #0 {
      n2 = flat-sequence {
        frame #0 {
          (unwired) FALSE ("Advance")
          # "Arrays that store the data across all advancements"
          # "Color Palette for Circles"
          # "Buttons"
          # "RGB for sensor image"
          # "RGB for selection image"
          n3 = Initialize Array("", 1 ("dimension size"), 100 ("dimension size")) -> (→"Region_array" →"Sensor_array":string[][])
          n4 = Initialize Array(0.0 ("element"), 1 ("dimension size"), 100 ("dimension size")) -> (→"X_array" →"Y_array":dbl[][])
          n5 = local write "Resample 2"(TRUE ("Resample")) -> ()
          n6 = local write "ErMsg 2"(FALSE ("ErMsg")) -> ()
          n7 = Build Array(u32 16711680 ("Green"), u32 15697664 ("Green 2"), u32 16772882 ("Green 5"), u32 8584960 ("Green 6"), u32 61382 ("Green 7"), u32 14847 ("Green 8"), u32 11534591 ("Green 9")) -> (w2:u32[])
          "Palette" <- w2
          n8 = local write "Resample"(TRUE ("Resample")) -> ()
          n9 = local write "ErMsg"(FALSE ("ErMsg")) -> ()
          n10 = Unbundle By Name("PerceptBtns") -> ()  [unwired: 9 out]
          n11 = Unbundle By Name("DscrptnBtns") -> ()  [unwired: 5 out]
          n12 = Index Array(array=w2, index=0) -> (element=→"CrcColor":u32)
          "RGB" <- dbl[] [] ("RGB Array")
          "RGBtbl" <- dbl[][] [] ("RGB Array")
          "Click" <- FALSE ("Resample")
          "RGB 2" <- dbl[] [] ("RGB Array")
          "RGBtbl 2" <- dbl[][] [] ("RGB Array")
          "Perception_array" <- string[] []
          "StepAdvnc" <- 0.0 ("StepAdvnc")
          "CursClck" <- dbl[] [] ("RGB Array")
          "Xcoord" <- dbl[] []
          "Ycoord" <- dbl[] []
          "Region" <- string[] []
          "Sensor" <- string[] []
          "Description_array" <- string[] []
          "SensorStr" <- "" ("SensorStr")
          "RegionStr" <- "" ("SensorStr")
        }
        frame #1 {
          # "Load look-up table for DEKA sensors"
          # "Load look-up table for selection regions"
          # "Selection Image"
          # "Sensor Image"
          n13 = global read "FeedbackDecode_Globals.vi" "FD_ResourcesDir"() -> (w45:path)
          n14 = global read "FeedbackDecode_Globals.vi" "FD_ResourcesDir"() -> (w48:path)
          n15 = global read "FeedbackDecode_Globals.vi" "FD_ResourcesDir"() -> (w42:path)
          n16 = global read "FeedbackDecode_Globals.vi" "FD_ResourcesDir"() -> (w51:path)
          n17 = Build Path(base path=w45, name or relative path="RGB_region_values.txt") -> (appended path=w43:path)
          n18 = Build Path(base path=w48, name or relative path="RightHand_sensor_colored.jpg") -> (appended path=w46:path)
          n19 = Build Path(base path=w42, name or relative path="RGB_sensor_values.txt") -> (appended path=w40:path)
          n20 = Build Path(base path=w51, name or relative path="RightHand_region_colored.jpg") -> (appended path=w49:path)
          "PPath2" <- w49
          n21 = Read from Text File(file (use dialog)=w43, count=-1) -> (text=w60:string)  [unwired: 2 in, 3 out]
          n22 = Read from Text File(file (use dialog)=w40, count=-1) -> (text=w74:string)  [unwired: 2 in, 3 out]
          n23 = call <vilib>:"Read JPEG File.vi"("path to JPEG file"=w49) -> ("image data"=w68:T5)  [unwired: 8 in, 2 out]
          n24 = call <vilib>:"Read JPEG File.vi"("path to JPEG file"=w46) -> ("image data"=w83:T5)  [unwired: 8 in, 2 out]
          n25 = call "Empty Picture"() -> ("empty picture"=w67:picture)
          n26 = call "Empty Picture"() -> ("empty picture"=w84:picture)
          n27 = Spreadsheet String To Array(format string="%d", spreadsheet string=w60, array type (2D Dbl)="Array 3") -> (array=w54:dbl[][])  [unwired: 1 in]
          n28 = Spreadsheet String To Array(format string="%d", spreadsheet string=w74, array type (2D Dbl)="Array 2") -> (array=w80:dbl[][])  [unwired: 1 in]
          n29 = call <vilib>:"Draw Flattened Pixmap.vi"("image data"=w68, "picture"=w67) -> ("new picture"=→"2D Picture 2":picture)  [unwired: 7 in]
          n30 = call <vilib>:"Draw Flattened Pixmap.vi"("image data"=w83, "picture"=w84) -> ("new picture"=→"2D Picture":picture)  [unwired: 7 in]
          n31 = Spreadsheet String To Array(format string="%s", spreadsheet string=w60, array type (2D Dbl)="Array 4") -> (array=→"RegionStr":string[][])  [unwired: 1 in]
          n32 = Spreadsheet String To Array(format string="%s", spreadsheet string=w74, array type (2D Dbl)="Array") -> (array=→"SensStr":string[][])  [unwired: 1 in]
          n33 = Index Array(array=w54, index (col) #1=2 ("disabled index (col)")) -> (element #1=w52:dbl[], element #2=w57:dbl[], element #3=w58:dbl[])  [unwired: 5 in]
          n34 = Index Array(array=w80, index (col) #1=2 ("disabled index (col)")) -> (element #1=w82:dbl[], element #2=w77:dbl[], element #3=w76:dbl[])  [unwired: 5 in]
          n35 = Build Array(w52, w57, w58) -> (w56:dbl[][])
          n36 = Build Array(w82, w77, w76) -> (w78:dbl[][])
          n37 = Transpose 2D Array(2D array=w56) -> (transposed array=w53:dbl[][])
          n38 = Transpose 2D Array(2D array=w78) -> (transposed array=w81:dbl[][])
          n39 = local write "RGBtbl 2"(w53) -> ()
          n40 = local write "RGBtbl"(w81) -> ()
        }
      }
    }
    frame #1 {
      # "DEKA Sensor Image"
      # "Selection Image"
      n41 = local read "2D Picture 2"() -> (w87:picture)
      n42 = local read "2D Picture"() -> (w86:picture)
      n43 = call <vilib>:"Picture to Pixmap.vi"("depth"=24, "picture"=w87) -> ("image data"=w91:T5)  [unwired: 8 in, 1 out]
      n44 = call <vilib>:"Picture to Pixmap.vi"("depth"=24, "picture"=w86) -> ("image data"=w94:T5)  [unwired: 8 in, 1 out]
      n45 = Unbundle By Name(w91) -> ("image"=w89:u8[], "Rectangle.right"=w88:i16)
      n46 = Unbundle By Name(w94) -> ("image"=w92:u8[], "Rectangle.right"=w93:i16)
      n47 = while {
        tunnel: w93 -> [w102]
        tunnel: w92 -> [w101]
        tunnel: w89 -> [w97]
        tunnel: w88 -> [w96]
        stop <- w98 stop-if-true
        n48 = event shown="[3] \"Submit\": Value Change" {
          selector: _ -> [_ _ _ _ _]
          dyn-events: _ -> [_ _ _ _ _]
          timeout: 100 -> [_ _ _ _ _]
          tunnel: w102 -> [_ w141 _ _ _]
          tunnel: w101 -> [_ w140 _ _ _]
          tunnel: w97 -> [_ w126 _ _ _]
          tunnel: w96 -> [_ w125 _ _ _]
          event Timeout {
            n49 = event-data() -> ()  [unwired: 1 in, 3 out]
            n50 = local write "Resample"(FALSE) -> ()
            n51 = local write "ErMsg"(FALSE) -> ()
          }
          event "2D Picture 2": Mouse Down? {
            # "Sensor"
            # "Region"
            # "X coord"
            # "Y coord"
            # "Draw Circle on Click"
            n52 = event-data() -> ("Coords"=w123:T3)  [unwired: 1 in]
            "Coords" <- w123
            n53 = local read "CrcColor"() -> (w118:u32)
            n54 = local read "2D Picture 2"() -> (w119:picture)
            n55 = Cluster To Array(cluster=w123) -> (array=w130:i32[])
            n56 = local write "Click"(TRUE ("Click")) -> ()
            n57 = call <vilib>:"Draw Circle by Radius.vi"("color(black)"=w118, "fill?(F)"=TRUE, "pixel center"=w123, "radius"=i16 5, "picture"=w119) -> ("new picture"=w134:picture)  [unwired: 6 in]
            n58 = local write "CursClck"(w130) -> ()
            n59 = property on="2D Picture 2" class="Pict"() -> ("Position"=w124:T6)  [unwired: 2 in, 2 out]
            n60 = property on="2D Picture" class="Pict"() -> ("Position"=w128:T6)  [unwired: 2 in, 2 out]
            n61 = Bundle(1, 0) -> (w132:cluster{i32, i32})  [unwired: 1 in]
            n62 = call <vilib>:"Draw Circle by Radius.vi"("pen"=w132, "pixel center"=w123, "radius"=i16 5, "picture"=w134) -> ("new picture"=w133:picture)  [unwired: 7 in]
            n63 = local write "2D Picture 2"(w133) -> ()
            n64 = while {
              tunnel: w123 -> [w152]
              tunnel: w125 -> [w157]
              tunnel: w126 -> [w170]
              tunnel: [w169] -> w122
              shift-right: [w150] -> _
              shift-left: -1 -> [w163]
              tunnel: w124 -> [w145]
              tunnel: [w143] -> w117
              tunnel: [w142] -> w121
              stop <- w159 stop-if-true
              # "Controls the case where no region\ncolor was identified (BW selection)"
              # "Terminates the check for a\nRGB near the click"
              # "Find the RGB values of the cursor location on the selection image"
              n65 = Add(x=w163, y=1) -> (x+y=w150:i32)
              "Count 2" <- w150
              n66 = case shown="3" w150 {
                tunnel: [w386 w389 w392 w395 w398 w401] -> w158
                frame 2 {
                  n67 = Bundle(0, 4) -> (w386:cluster{i32, i32})  [unwired: 1 in]
                }
                frame 3 {
                  n68 = Bundle(-4, 0) -> (w389:cluster{i32, i32})  [unwired: 1 in]
                }
                frame 4 {
                  n69 = Bundle(0, -4) -> (w392:cluster{i32, i32})  [unwired: 1 in]
                }
                frame Default {
                  n70 = Bundle(0, 0) -> (w395:cluster{i32, i32})  [unwired: 1 in]
                }
                frame 0 {
                  n71 = Bundle(0, 0) -> (w398:cluster{i32, i32})  [unwired: 1 in]
                }
                frame 1 {
                  n72 = Bundle(4, 0) -> (w401:cluster{i32, i32})  [unwired: 1 in]
                }
              }
              n73 = local read "RGBtbl 2"() -> (w151:dbl[][])
              n74 = Add(x=w152, y=w158) -> (x+y=w161:T3)
              n75 = Subtract(x=w161, y=w145) -> (x-y=w144:T3)
              n76 = Cluster To Array(cluster=w144) -> (array=w143:i32[])
              n77 = Unbundle By Name(w144) -> ("Horizontal"=w155:i32, "Vertical"=w171:i32)
              n78 = Multiply(x=w157, y=w171) -> (x*y=w177:i32)
              n79 = Add(x=-3, y=w155) -> (x+y=w156:i32)
              n80 = Add(x=w156, y=w177) -> (x+y=w176:i32)
              n81 = Multiply(x=3, y=w176) -> (x*y=w174:i32)
              n82 = Increment(x=w174) -> (x+1=w173:i32)
              n83 = Increment(x=w173) -> (x+1=w172:i32)
              n84 = Index Array(array=w170, index #1=w174, index #2=w173, index #3=w172) -> (element #1=w167:u8, element #2=w166:u8, element #3=w165:u8)
              n85 = Insert Into Array(array=dbl[] [] ("Horizontal"), new element #1=w167, new element #2=w166, new element #3=w165) -> (w147:dbl[])  [unwired: 1 in]
              n86 = mathscript code="BW = 0;\nmx=0;\nErMsg = 1;\ny(:,1) = abs(RGBtbl(:,1) - RGB(1));\ny(:,2) = abs(RGBtbl(:,2) - RGB(2));\ny(:,3) = abs(RGBtbl(:,3) - RGB(3));\nif Cnt > 4\n     BW=0;\n     ErMsg = 1;\nelseif min(sum(y,2))<10;\n     [mn,mx] = min(sum(y,2));\n     BW = 0;\nelse \n     BW = 1;\nend"("RGBtbl"=w151, "RGB"=w147, "Cnt"=w150) -> ("BW"=w149:i32, "ErMsg"=w148:i32, "mx"=w146:i32)  [unwired: 1 in, 1 out]
              n87 = Equal?(x=w148, y=0.0) -> (x = y?=w153:bool)
              "ErMsg 2" <- w153
              n88 = Equal?(x=w149, y=0.0) -> (x = y?=w159:bool)
              "Resample 2" <- w159
              n89 = case shown="False" w153 {
                tunnel: w146 -> [w380 _]
                tunnel: [w379 "None" ("StrSensor")] -> w142
                frame False {
                  n90 = local read "RegionStr"() -> (w383:string[][])
                  n91 = Subtract(x=w380, y=u8 1) -> (x-y=w382:i32)
                  n92 = Index Array(array=w383, index (row)=w382, index (col)=5 ("disabled index (col)")) -> (element=w379:string)
                }
                frame True {
                }
              }
              n93 = call <vilib>:"RGB to Color.vi"("B"=w165, "G"=w166, "R"=w167) -> ("Color"=w169:u32)
              n94 = local write "RGB 2"(w147) -> ()
            }
            "Output Color" <- w122
            n95 = while {
              tunnel: w123 -> [w412]
              tunnel: w141 -> [w417]
              tunnel: w140 -> [w431]
              tunnel: [w430] -> _
              shift-right: [w410] -> _
              shift-left: -1 -> [w424]
              tunnel: w128 -> [w405]
              tunnel: [w404] -> w120
              stop <- w419 stop-if-true
              # "Controls the case where no\nsensor color was identified (BW)"
              # "Terminates the check for a\nRGB near the click"
              # "Find the RGB values of the cursor location to identify the DEKA sensor"
              n96 = Add(x=w424, y=1) -> (x+y=w410:i32)
              "Count" <- w410
              n97 = case shown="3" w410 {
                tunnel: [w647 w650 w653 w656 w659 w662] -> w418
                frame 2 {
                  n98 = Bundle(0, 10) -> (w647:cluster{i32, i32})  [unwired: 1 in]
                }
                frame 3 {
                  n99 = Bundle(-10, 0) -> (w650:cluster{i32, i32})  [unwired: 1 in]
                }
                frame 4 {
                  n100 = Bundle(0, -10) -> (w653:cluster{i32, i32})  [unwired: 1 in]
                }
                frame Default {
                  n101 = Bundle(0, 0) -> (w656:cluster{i32, i32})  [unwired: 1 in]
                }
                frame 0 {
                  n102 = Bundle(0, 0) -> (w659:cluster{i32, i32})  [unwired: 1 in]
                }
                frame 1 {
                  n103 = Bundle(10, 0) -> (w662:cluster{i32, i32})  [unwired: 1 in]
                }
              }
              n104 = local read "RGBtbl"() -> (w411:dbl[][])
              n105 = Add(x=w412, y=w418) -> (x+y=w421:T3)
              n106 = Subtract(x=w421, y=w405) -> (x-y=w422:T3)
              n107 = Unbundle By Name(w422) -> ("Horizontal"=w415:i32, "Vertical"=w432:i32)
              n108 = Multiply(x=w417, y=w432) -> (x*y=w438:i32)
              n109 = Add(x=-3, y=w415) -> (x+y=w416:i32)
              n110 = Add(x=w416, y=w438) -> (x+y=w437:i32)
              n111 = Multiply(x=3, y=w437) -> (x*y=w435:i32)
              n112 = Increment(x=w435) -> (x+1=w434:i32)
              n113 = Increment(x=w434) -> (x+1=w433:i32)
              n114 = Index Array(array=w431, index #1=w435, index #2=w434, index #3=w433) -> (element #1=w428:u8, element #2=w427:u8, element #3=w426:u8)
              n115 = Insert Into Array(array=dbl[] [] ("Horizontal"), new element #1=w428, new element #2=w427, new element #3=w426) -> (w407:dbl[])  [unwired: 1 in]
              n116 = mathscript code="BW = 0;\nmx=0;\nErMsg = 1;\ny(:,1) = abs(RGBtbl(:,1) - RGB(1));\ny(:,2) = abs(RGBtbl(:,2) - RGB(2));\ny(:,3) = abs(RGBtbl(:,3) - RGB(3));\nif Cnt > 4\n     BW=0;\n     ErMsg = 1;\nelseif min(sum(y,2))<10;\n     [mn,mx] = min(sum(y,2));\n     BW = 0;\nelse \n     BW = 1;\nend"("RGBtbl"=w411, "RGB"=w407, "Cnt"=w410) -> ("BW"=w409:i32, "ErMsg"=w408:i32, "mx"=w406:i32)  [unwired: 1 in, 1 out]
              n117 = Equal?(x=w408, y=0.0) -> (x = y?=w413:bool)
              "ErMsg" <- w413
              n118 = Equal?(x=w409, y=0.0) -> (x = y?=w419:bool)
              "Resample" <- w419
              n119 = case shown="False" w413 {
                tunnel: w406 -> [w641 _]
                tunnel: [w640 "None" ("StrSensor")] -> w404
                frame False {
                  n120 = local read "SensStr"() -> (w644:string[][])
                  n121 = Subtract(x=w641, y=u8 1) -> (x-y=w643:i32)
                  n122 = Index Array(array=w644, index (row)=w643, index (col)=5 ("disabled index (col)")) -> (element=w640:string)
                }
                frame True {
                }
              }
              n123 = call <vilib>:"RGB to Color.vi"("B"=w426, "G"=w427, "R"=w428) -> ("Color"=w430:u32)
              n124 = local write "RGB"(w407) -> ()
            }
            n125 = Split 1D Array(array=w117, index=1) -> (first subarray=w114:i32[], second subarray=w116:i32[])
            n126 = local read "Xcoord"() -> (w113:dbl[])
            n127 = Insert Into Array(array=w113, new element=w114) -> (w110:dbl[])  [unwired: 1 in]
            n128 = local write "Xcoord"(w110) -> ()
            n129 = local read "Ycoord"() -> (w111:dbl[])
            n130 = Insert Into Array(array=w111, new element=w116) -> (w112:dbl[])  [unwired: 1 in]
            n131 = local write "Ycoord"(w112) -> ()
            n132 = local read "Sensor"() -> (w107:string[])
            n133 = local read "Region"() -> (w109:string[])
            n134 = Insert Into Array(array=w107, new element=w120) -> (w106:string[])  [unwired: 1 in]
            n135 = local write "Sensor"(w106) -> ()
            n136 = Insert Into Array(array=w109, new element=w121) -> (w108:string[])  [unwired: 1 in]
            n137 = local write "Region"(w108) -> ()
            n138 = event-data() -> ()  [unwired: 2 in, 1 out]
          }
          event "Advance": Value Change {
            # "Insert pushed Perception Button into the array\nOnly 1 button is pushed so only 1 string for each row of array"
            n139 = event-data() -> ()  [unwired: 1 in, 6 out]
            n140 = flat-sequence {
              frame #0 {
                w700 = ""
                w733 = ""
                # "Inserts DEKA sensor array from multiple clicks into the 2D array"
                # "Inserts Regions array from multiple clicks into the 2D array"
                # "Inserts X and Y array of clicks into the 2D array"
                # "Insert the Pushed Description Buttons into the array as a array of strings for each row (type of percept)"
                n141 = local read "DscrptnBtns"() -> (w671:T1)
                n142 = local read "PerceptBtns"() -> (w752:T2)
                n143 = Unbundle By Name(w671) -> ("2afc 3"=w670:cluster{"Stationary":bool, "Migratory":bool}, "2afc 2"=w669:cluster{"Natural":bool, "Unnatural":bool}, "2afc 4"=w668:cluster{"Confined":bool, "Spread":bool}, "2afc 1"=w667:cluster{"Intermittent":bool, "Sustained":bool}, "2afc 0"=w666:cluster{"Deep":bool, "Surface":bool})
                n144 = Unbundle By Name(w752) -> ("Buzzing"=w751:bool, "Pressure"=w750:bool, "Tapping"=w749:bool, "None"=w748:bool, "Flutter"=w747:bool, "Vibration"=w743:bool, "Pain"=w746:bool, "Tightening"=w745:bool, "Movement"=w744:bool)
                n145 = Unbundle By Name(w670) -> ("Stationary"=w720:bool, "Migratory"=w719:bool)
                n146 = Unbundle By Name(w669) -> ("Natural"=w718:bool, "Unnatural"=w717:bool)
                n147 = Unbundle By Name(w668) -> ("Confined"=w716:bool, "Spread"=w715:bool)
                n148 = Unbundle By Name(w666) -> ("Deep"=w712:bool, "Surface"=w711:bool)
                n149 = Unbundle By Name(w667) -> ("Intermittent"=w714:bool, "Sustained"=w713:bool)
                n150 = Select(t="Buzzing", s=w751, f=w733) -> (s? t:f=w732:string)
                n151 = Select(t="Pressure", s=w750, f=w733) -> (s? t:f=w731:string)
                n152 = Select(t="Tapping", s=w749, f=w733) -> (s? t:f=w730:string)
                n153 = Select(t="Flutter", s=w747, f=w733) -> (s? t:f=w728:string)
                n154 = Select(t="Vibration", s=w743, f=w733) -> (s? t:f=w727:string)
                n155 = Select(t="Movement", s=w744, f=w733) -> (s? t:f=w726:string)
                n156 = Select(t="Tightening", s=w745, f=w733) -> (s? t:f=w724:string)
                n157 = Select(t="Pain", s=w746, f=w733) -> (s? t:f=w725:string)
                n158 = Select(t="None", s=w748, f=w733) -> (s? t:f=w729:string)
                n159 = Select(t="'Stationary';", s=w720, f=w700) -> (s? t:f=w685:string)
                n160 = Select(t="'Migratory';", s=w719, f=w700) -> (s? t:f=w679:string)
                n161 = Select(t="'Natural';", s=w718, f=w700) -> (s? t:f=w678:string)
                n162 = Select(t="'Unnatural';", s=w717, f=w700) -> (s? t:f=w680:string)
                n163 = Select(t="'Confined';", s=w716, f=w700) -> (s? t:f=w683:string)
                n164 = Select(t="'Spread';", s=w715, f=w700) -> (s? t:f=w682:string)
                n165 = Select(t="'Intermittent';", s=w714, f=w700) -> (s? t:f=w681:string)
                n166 = Select(t="'Sustained';", s=w713, f=w700) -> (s? t:f=w677:string)
                n167 = Select(t="'Deep';", s=w712, f=w700) -> (s? t:f=w676:string)
                n168 = Select(t="'Surface';", s=w711, f=w700) -> (s? t:f=w675:string)
                n169 = local read "Perception_array"() -> (w723:string[])
                n170 = Concatenate Strings(w732, w731, w730, w729, w728, w727, w726, w725, w724) -> (w722:string)
                n171 = local read "Description_array"() -> (w673:string[])
                n172 = Concatenate Strings("{" ("string"), w685, w679, w678, w680, w683, w682, w681, w677, w676, w675, "}" ("string")) -> (w672:string)
                n173 = Insert Into Array(array=w673, new element=w672) -> (w674:string[])  [unwired: 1 in]
                n174 = Insert Into Array(array=w723, new element=w722) -> (w721:string[])  [unwired: 1 in]
                n175 = local write "Perception_array"(w721) -> ()
                n176 = local write "Description_array"(w674) -> ()
                n177 = local read "Region_array"() -> (w692:string[][])
                n178 = local read "Sensor_array"() -> (w691:string[][])
                n179 = local read "Xcoord"() -> (w697:dbl[])
                n180 = local read "Ycoord"() -> (w686:dbl[])
                n181 = local read "Sensor"() -> (w687:string[])
                n182 = local read "StepAdvnc"() -> (w689:dbl)
                n183 = local read "X_array"() -> (w699:dbl[][])
                n184 = local read "Y_array"() -> (w695:dbl[][])
                n185 = local read "Region"() -> (w694:string[])
                n186 = Insert Into Array(array=w699, new element=w697) -> (w698:dbl[][])  [unwired: 2 in]
                n187 = Insert Into Array(array=w695, new element=w686) -> (w696:dbl[][])  [unwired: 2 in]
                n188 = Insert Into Array(array=w691, new element=w687) -> (w690:string[][])  [unwired: 2 in]
                n189 = Insert Into Array(array=w692, new element=w694) -> (w693:string[][])  [unwired: 2 in]
                n190 = Increment(x=w689) -> (x+1=w688:dbl)
                n191 = local write "X_array"(w698) -> ()
                n192 = local write "Y_array"(w696) -> ()
                n193 = local write "Region_array"(w693) -> ()
                n194 = local write "Sensor_array"(w690) -> ()
                n195 = local write "StepAdvnc"(w688) -> ()
              }
              frame #1 {
                # "Change the color of the circle to draw next"
                # "Reset all the buttons and Temp variables"
                n196 = local read "StepAdvnc"() -> (w756:dbl)
                n197 = local read "Palette"() -> (w765:u32[])
                n198 = local write "PerceptBtns"(T4 {"Motion"=FALSE, "Pressure"=FALSE, "Tapping"=FALSE, "None"=FALSE, "Flutter"=FALSE, "Vibration"=FALSE, "Pain"=FALSE, "Tightening"=FALSE, "Movement"=FALSE} ("PerceptBtns")) -> ()
                n199 = local write "DscrptnBtns"(T1 {"2afc 3"={"Stationary"=FALSE, "Migratory"=FALSE}, "2afc 2"={"Natural"=FALSE, "Unnatural"=FALSE}, "2afc 4"={"Confined"=FALSE, "Spread"=FALSE}, "2afc 1"={"Intermittent"=FALSE, "Sustained"=FALSE}, "2afc 0"={"Deep"=FALSE, "Surface"=FALSE}} ("DscrptnBtns")) -> ()
                n200 = local write "Region"(string[] [] ("Region")) -> ()
                n201 = local write "Sensor"(string[] [] ("Sensor")) -> ()
                n202 = local write "Advance"(FALSE ("Advance")) -> ()
                n203 = local write "Xcoord"(dbl[] [] ("Xcoord")) -> ()
                n204 = local write "Ycoord"(dbl[] [] ("Xcoord")) -> ()
                n205 = local write "Click"(FALSE ("Submit")) -> ()
                n206 = Index Array(array=w765, index=w756) -> (element=w766:u32)
                n207 = local write "CrcColor"(w766) -> ()
                n208 = local write "CursClck"(dbl[] [] ("RGB Array")) -> ()
                n209 = local write "Resample"(TRUE ("Resample")) -> ()
                n210 = local write "ErMsg"(FALSE ("ErMsg")) -> ()
              }
            }
          }
          event "Submit": Value Change {
            # "This frame is in case the continue button is not pushed before submit"
            # "This event will send the string to the main FeedbackDecode.vi to store, and reset the variables/image etc..."
            n211 = event-data() -> ()  [unwired: 1 in, 6 out]
            n212 = flat-sequence {
              frame #0 {
                n213 = local read "Advance"() -> (w767:bool)
                n214 = case shown="False" w767 {
                  frame False {
                    w803 = ""
                    w836 = ""
                    # "Inserts DEKA sensor array from multiple clicks into the 2D array"
                    # "Inserts Regions array from multiple clicks into the 2D array"
                    # "Inserts X and Y array of clicks into the 2D array"
                    # "Insert the Pushed Description Buttons into the array as a array of strings for each row (type of percept)"
                    # "Insert pushed Perception Button into the array\nOnly 1 button is pushed so only 1 string for each row of array"
                    n215 = local read "DscrptnBtns"() -> (w774:T1)
                    n216 = local read "PerceptBtns"() -> (w855:T2)
                    n217 = Unbundle By Name(w774) -> ("2afc 3"=w773:cluster{"Stationary":bool, "Migratory":bool}, "2afc 2"=w772:cluster{"Natural":bool, "Unnatural":bool}, "2afc 4"=w771:cluster{"Confined":bool, "Spread":bool}, "2afc 1"=w770:cluster{"Intermittent":bool, "Sustained":bool}, "2afc 0"=w769:cluster{"Deep":bool, "Surface":bool})
                    n218 = Unbundle By Name(w855) -> ("Buzzing"=w854:bool, "Pressure"=w853:bool, "Tapping"=w852:bool, "None"=w851:bool, "Flutter"=w850:bool, "Vibration"=w846:bool, "Pain"=w849:bool, "Tightening"=w848:bool, "Movement"=w847:bool)
                    n219 = Unbundle By Name(w773) -> ("Stationary"=w823:bool, "Migratory"=w822:bool)
                    n220 = Unbundle By Name(w772) -> ("Natural"=w821:bool, "Unnatural"=w820:bool)
                    n221 = Unbundle By Name(w771) -> ("Confined"=w819:bool, "Spread"=w818:bool)
                    n222 = Unbundle By Name(w769) -> ("Deep"=w815:bool, "Surface"=w814:bool)
                    n223 = Unbundle By Name(w770) -> ("Intermittent"=w817:bool, "Sustained"=w816:bool)
                    n224 = Select(t="Buzzing", s=w854, f=w836) -> (s? t:f=w835:string)
                    n225 = Select(t="Pressure", s=w853, f=w836) -> (s? t:f=w834:string)
                    n226 = Select(t="Tapping", s=w852, f=w836) -> (s? t:f=w833:string)
                    n227 = Select(t="Flutter", s=w850, f=w836) -> (s? t:f=w831:string)
                    n228 = Select(t="Vibration", s=w846, f=w836) -> (s? t:f=w830:string)
                    n229 = Select(t="Movement", s=w847, f=w836) -> (s? t:f=w829:string)
                    n230 = Select(t="Tightening", s=w848, f=w836) -> (s? t:f=w827:string)
                    n231 = Select(t="Pain", s=w849, f=w836) -> (s? t:f=w828:string)
                    n232 = Select(t="None", s=w851, f=w836) -> (s? t:f=w832:string)
                    n233 = Select(t="'Stationary';", s=w823, f=w803) -> (s? t:f=w788:string)
                    n234 = Select(t="'Migratory';", s=w822, f=w803) -> (s? t:f=w782:string)
                    n235 = Select(t="'Natural';", s=w821, f=w803) -> (s? t:f=w781:string)
                    n236 = Select(t="'Unnatural';", s=w820, f=w803) -> (s? t:f=w783:string)
                    n237 = Select(t="'Confined';", s=w819, f=w803) -> (s? t:f=w786:string)
                    n238 = Select(t="'Spread';", s=w818, f=w803) -> (s? t:f=w785:string)
                    n239 = Select(t="'Intermittent';", s=w817, f=w803) -> (s? t:f=w784:string)
                    n240 = Select(t="'Sustained';", s=w816, f=w803) -> (s? t:f=w780:string)
                    n241 = Select(t="'Deep';", s=w815, f=w803) -> (s? t:f=w779:string)
                    n242 = Select(t="'Surface';", s=w814, f=w803) -> (s? t:f=w778:string)
                    n243 = local read "Perception_array"() -> (w826:string[])
                    n244 = Concatenate Strings(w835, w834, w833, w832, w831, w830, w829, w828, w827) -> (w825:string)
                    n245 = local read "Description_array"() -> (w776:string[])
                    n246 = Concatenate Strings("{" ("string"), w788, w782, w781, w783, w786, w785, w784, w780, w779, w778, "}" ("string")) -> (w775:string)
                    n247 = Insert Into Array(array=w826, new element=w825) -> (w824:string[])  [unwired: 1 in]
                    n248 = local write "Perception_array"(w824) -> ()
                    n249 = Insert Into Array(array=w776, new element=w775) -> (w777:string[])  [unwired: 1 in]
                    n250 = local write "Description_array"(w777) -> ()
                    n251 = local read "Region_array"() -> (w795:string[][])
                    n252 = local read "Sensor_array"() -> (w794:string[][])
                    n253 = local read "Xcoord"() -> (w800:dbl[])
                    n254 = local read "Ycoord"() -> (w789:dbl[])
                    n255 = local read "StepAdvnc"() -> (w792:dbl)
                    n256 = local read "Sensor"() -> (w790:string[])
                    n257 = local read "X_array"() -> (w802:dbl[][])
                    n258 = local read "Y_array"() -> (w798:dbl[][])
                    n259 = local read "Region"() -> (w797:string[])
                    n260 = Insert Into Array(array=w802, new element=w800) -> (w801:dbl[][])  [unwired: 2 in]
                    n261 = Insert Into Array(array=w798, new element=w789) -> (w799:dbl[][])  [unwired: 2 in]
                    n262 = Insert Into Array(array=w794, new element=w790) -> (w793:string[][])  [unwired: 2 in]
                    n263 = Increment(x=w792) -> (x+1=w791:dbl)
                    n264 = Insert Into Array(array=w795, new element=w797) -> (w796:string[][])  [unwired: 2 in]
                    n265 = local write "X_array"(w801) -> ()
                    n266 = local write "Y_array"(w799) -> ()
                    n267 = local write "Region_array"(w796) -> ()
                    n268 = local write "Sensor_array"(w793) -> ()
                    n269 = local write "StepAdvnc"(w791) -> ()
                  }
                  frame True {
                  }
                }
              }
              frame #1 {
                n270 = local read "Description_array"() -> (w862:string[])
                n271 = local read "Perception_array"() -> (w863:string[])
                n272 = local read "Region_array"() -> (w858:string[][])
                n273 = local read "Sensor_array"() -> (w859:string[][])
                n274 = local read "X_array"() -> (w861:dbl[][])
                n275 = local read "Y_array"() -> (w860:dbl[][])
                n276 = call "FeedbackDecode_ParsePickROIStr.vi"("Perception_array"=w863, "Description_array"=w862, "X_array"=w861, "Y_array"=w860, "Sensor_array"=w859, "Region_array"=w858) -> ("ROIStr"=w857:string)  [unwired: 13 in]
                "PickROIStr" <- w857
                n277 = property on="Property Node" class="Str"(reference="RespStrRef", "Val(Sgnl)"=w857) -> ()  [unwired: 1 in, 2 out]
              }
              frame #2 {
                w864 = FALSE ("Submit")
                # "Draw a clean image"
                # "Reset the arrays"
                # "Reset the color of the circle"
                # "Reset all the buttons and Temp variables"
                n278 = local write "Resample 2"(TRUE ("Resample")) -> ()
                n279 = local write "ErMsg 2"(FALSE ("ErMsg")) -> ()
                n280 = local read "Palette"() -> (w894:u32[])
                n281 = local write "Resample"(TRUE ("Resample")) -> ()
                n282 = local write "ErMsg"(FALSE ("ErMsg")) -> ()
                n283 = local read "PPath2"() -> (w878:path)
                n284 = local write "PerceptBtns"(T4 {"Motion"=FALSE, "Pressure"=FALSE, "Tapping"=FALSE, "None"=FALSE, "Flutter"=FALSE, "Vibration"=FALSE, "Pain"=FALSE, "Tightening"=FALSE, "Movement"=FALSE} ("PerceptBtns")) -> ()
                n285 = local write "DscrptnBtns"(T1 {"2afc 3"={"Stationary"=FALSE, "Migratory"=FALSE}, "2afc 2"={"Natural"=FALSE, "Unnatural"=FALSE}, "2afc 4"={"Confined"=FALSE, "Spread"=FALSE}, "2afc 1"={"Intermittent"=FALSE, "Sustained"=FALSE}, "2afc 0"={"Deep"=FALSE, "Surface"=FALSE}} ("DscrptnBtns")) -> ()
                n286 = local write "Region"(string[] [] ("Region")) -> ()
                n287 = local write "Sensor"(string[] [] ("Sensor")) -> ()
                n288 = local write "Advance"(FALSE ("Advance")) -> ()
                n289 = local write "Xcoord"(dbl[] [] ("Xcoord")) -> ()
                n290 = local write "Xcoord"(dbl[] [] ("Xcoord")) -> ()
                n291 = local write "Click"(FALSE ("Submit")) -> ()
                n292 = local read "2D Picture 2"() -> (w877:picture)
                n293 = Index Array(array=w894, index=0) -> (element=w895:u32)
                n294 = call <vilib>:"Read JPEG File.vi"("path to JPEG file"=w878) -> ("image data"=w875:T5)  [unwired: 8 in, 2 out]
                n295 = local write "CrcColor"(w895) -> ()
                n296 = local write "CursClck"(dbl[] [] ("RGB Array")) -> ()
                n297 = local write "Advance"(w864) -> ()
                n298 = local write "Submit"(w864) -> ()
                n299 = call <vilib>:"Draw Flattened Pixmap.vi"("image data"=w875, "picture"=w877) -> ("new picture"=w876:picture)  [unwired: 7 in]
                n300 = local write "2D Picture 2"(w876) -> ()
                n301 = Initialize Array("", 1 ("dimension size"), 100 ("dimension size")) -> (w867:string[][])
                n302 = Initialize Array(0.0 ("element"), 1 ("dimension size"), 100 ("dimension size")) -> (w868:dbl[][])
                n303 = local write "Perception_array"(string[] [] ("Perception_array")) -> ()
                n304 = local write "Description_array"(string[] [] ("Description_array")) -> ()
                n305 = local write "Region_array"(w867) -> ()
                n306 = local write "Sensor_array"(w867) -> ()
                n307 = local write "StepAdvnc"(0.0 ("StepAdvnc")) -> ()
                n308 = local write "X_array"(w868) -> ()
                n309 = local write "Y_array"(w868) -> ()
              }
            }
          }
          event "ClearRsp": Value Change {
            w906 = FALSE ("Submit")
            # "Draw a clean image"
            # "Reset the arrays"
            # "Reset the color of the circle"
            # "Reset all the buttons and Temp variables"
            n310 = event-data() -> ()  [unwired: 1 in, 6 out]
            n311 = local write "Resample 2"(TRUE ("Resample")) -> ()
            n312 = local write "ErMsg 2"(FALSE ("ErMsg")) -> ()
            n313 = local read "Palette"() -> (w926:u32[])
            n314 = local write "Resample"(TRUE ("Resample")) -> ()
            n315 = local write "ErMsg"(FALSE ("ErMsg")) -> ()
            n316 = local read "PPath2"() -> (w910:path)
            n317 = local write "PerceptBtns"(T4 {"Motion"=FALSE, "Pressure"=FALSE, "Tapping"=FALSE, "None"=FALSE, "Flutter"=FALSE, "Vibration"=FALSE, "Pain"=FALSE, "Tightening"=FALSE, "Movement"=FALSE} ("PerceptBtns")) -> ()
            n318 = local write "DscrptnBtns"(T1 {"2afc 3"={"Stationary"=FALSE, "Migratory"=FALSE}, "2afc 2"={"Natural"=FALSE, "Unnatural"=FALSE}, "2afc 4"={"Confined"=FALSE, "Spread"=FALSE}, "2afc 1"={"Intermittent"=FALSE, "Sustained"=FALSE}, "2afc 0"={"Deep"=FALSE, "Surface"=FALSE}} ("DscrptnBtns")) -> ()
            n319 = local write "Region"(string[] [] ("Region")) -> ()
            n320 = local write "Sensor"(string[] [] ("Sensor")) -> ()
            n321 = local write "Advance"(FALSE ("Advance")) -> ()
            n322 = local write "Xcoord"(dbl[] [] ("Xcoord")) -> ()
            n323 = local write "Xcoord"(dbl[] [] ("Xcoord")) -> ()
            n324 = local write "Click"(FALSE ("Submit")) -> ()
            n325 = local read "2D Picture 2"() -> (w909:picture)
            n326 = Index Array(array=w926, index=0) -> (element=w927:u32)
            n327 = call <vilib>:"Read JPEG File.vi"("path to JPEG file"=w910) -> ("image data"=w907:T5)  [unwired: 8 in, 2 out]
            n328 = local write "CrcColor"(w927) -> ()
            n329 = local write "CursClck"(dbl[] [] ("RGB Array")) -> ()
            n330 = local write "ClearRsp"(w906) -> ()
            n331 = local write "Submit"(w906) -> ()
            n332 = call <vilib>:"Draw Flattened Pixmap.vi"("image data"=w907, "picture"=w909) -> ("new picture"=w908:picture)  [unwired: 7 in]
            n333 = local write "2D Picture 2"(w908) -> ()
            n334 = Initialize Array("", 1 ("dimension size"), 100 ("dimension size")) -> (w898:string[][])
            n335 = Initialize Array(0.0 ("element"), 1 ("dimension size"), 100 ("dimension size")) -> (w899:dbl[][])
            n336 = local write "Perception_array"(string[] [] ("Perception_array")) -> ()
            n337 = local write "Region_array"(w898) -> ()
            n338 = local write "Sensor_array"(w898) -> ()
            n339 = local write "StepAdvnc"(0.0 ("StepAdvnc")) -> ()
            n340 = local write "X_array"(w899) -> ()
            n341 = local write "Y_array"(w899) -> ()
            n342 = local write "Description_array"(string[] [] ("Description_array")) -> ()
          }
        }
        n343 = global read "FeedbackDecode_Globals.vi" "FD_Stop"() -> (w99:bool)
        n344 = local read "Abort"() -> (w100:bool)
        n345 = Or(x=w100, y=w99) -> (x .or. y?=w98:bool)
      }
    }
    frame #2 {
      n346 = disable-structure shown="Disabled" {
        frame Disabled {
          n347 = control-ref of="This VI"() -> (w929:refnum<vi>)
          n348 = property class="VI"(reference=w929) -> (reference out=w930:refnum<vi>, "FP.State"=w931:T7)  [unwired: 1 in, 1 out]
          n349 = case shown="\"Standard\", Default" w931 {
            tunnel: w930 -> [_ w932]
            frame "Closed" {
            }
            frame "Standard", Default {
              n350 = invoke class="VI" method="FP.Close"(reference=w932) -> ()  [unwired: 2 in, 3 out]
            }
          }
        }
        frame Enabled {
        }
      }
      n351 = local write "Abort"(FALSE ("Abort")) -> ()
    }
  }
